vi "Vision_Left_R3.2.vi"() -> ()   [LabVIEW 2015]
uses:
  <vilib>/vision/Pattern Matching.llb/IMAQ Curve Parameters.ctl
  <vilib>/vision/Pattern Matching.llb/IMAQ Match Range Setting.ctl
  <vilib>/userdefined/High Color/IMAQdx.ctl
  <vilib>/vision/driver/NI_Vision_Acquisition_Software.lvlib
  <vilib>/vision/NI_Vision_Development_Module.lvlib
panel:
  in  "Range 0 Default\nSetting Values":T1={"Min Scale"=50.0, "Max Scale"=160.0, "Min Score"=850.0, "Lower Transition Scale"=55.0, "Upper Transition Scale"=200.0, "ROI Vertical"=4.5, "ROI Horizontal"=2.5, "Scale Cushion"=7.0, "Curve Parameters"={"Min Length"=20, "Row Search Step"=15, "Col Search Step"=15}, "Beacon Cushion (px)"=3.0, "Max Scale Diff\nfrom Main"=50.0}
  in  "Range 0 Templates":T2={"Sub - 2 File Path"=path "/home/lvuser/Beacon_Templates/Range_0/Range 0.png", "Sub Beacon Template File Path - ARRAY"=[path "/home/lvuser/Beacon_Templates/Range_1/Sub 0 - Range 1.png", path "/home/lvuser/Beacon_Templates/Range_1/Sub 1 - Range 1.png", path "/home/lvuser/Beacon_Templates/Range_1/Sub 2 - Range 1.png", path "/home/lvuser/Beacon_Templates/Range_1/Sub 3 - Range 1.png", path "/home/lvuser/Beacon_Templates/Range_1/Sub 4 - Range 1.png"]}
  in  "Correlation Score Threhsold (Range 0)":sgl=750.0
  in  "stop":bool
  in  "select (true= use advanced features\nfase= dont use)":bool
  in  "Range 3 Default\nSetting Values":T1={"Min Scale"=50.0, "Max Scale"=130.0, "Min Score"=800.0, "Lower Transition Scale"=1.0, "Upper Transition Scale"=120.0, "ROI Vertical"=3.5, "ROI Horizontal"=4.0, "Scale Cushion"=15.0, "Curve Parameters"={"Min Length"=2, "Row Search Step"=5, "Col Search Step"=5}, "Beacon Cushion (px)"=3.0, "Max Scale Diff\nfrom Main"=10.0}
  in  "Range 2 Default\nSetting Values":T1={"Min Scale"=75.0, "Max Scale"=130.0, "Min Score"=800.0, "Lower Transition Scale"=70.0, "Upper Transition Scale"=115.0, "ROI Vertical"=2.8, "ROI Horizontal"=4.0, "Scale Cushion"=17.0, "Curve Parameters"={"Min Length"=10, "Row Search Step"=10, "Col Search Step"=10}, "Beacon Cushion (px)"=7.0, "Max Scale Diff\nfrom Main"=20.0}
  in  "No Lock Default\nSetting Values":T3={"Min Scale"=25.0, "Max Scale"=125.0, "Min Score"=750.0, "Lower Transition Scale"=35.0, "Upper Transition Scale"=250.0, "ROI Vertical"=15.0, "ROI Horizontal"=15.0, "Scale Cushion"=15.0, "Curve Parameters"={"Min Length"=5, "Row Search Step"=10, "Col Search Step"=10}, "Scale Cushion 2"=15.0, "Max Scale Diff\nfrom Main"=15.0}
  in  "ROI Decay Factor (px)":dbl=50.0
  in  "ROBOT STATE\n(fwd, bwd, neither) 2":i32
  in  "Score Decay \nFactor 2":dbl=50.0
  in  "Range 1 Default\nSetting Values":T1={"Min Scale"=30.0, "Max Scale"=100.0, "Min Score"=800.0, "Lower Transition Scale"=35.0, "Upper Transition Scale"=67.0, "ROI Vertical"=0.75, "ROI Horizontal"=5.0, "Scale Cushion"=20.0, "Curve Parameters"={"Min Length"=15, "Row Search Step"=15, "Col Search Step"=15}, "Beacon Cushion (px)"=25.0, "Max Scale Diff\nfrom Main"=25.0}
  out "Next Template":T4(ring)=enum."Range 3"
  out "Current Template":T4(ring)=enum."Range 3"
  in  "Initial Template":T4(ring)
  in  "Range 3 Templates":T2={"Sub - 2 File Path"=path "/home/lvuser/Beacon_Templates/Range_3/5 Beacons - Range 3.png", "Sub Beacon Template File Path - ARRAY"=[path "/home/lvuser/Beacon_Templates/Range_3/Sub 0 - Range 3.png", path "/home/lvuser/Beacon_Templates/Range_3/Sub 1 - Range 3.png", path "/home/lvuser/Beacon_Templates/Range_3/Sub 2 - Range 3.png", path "/home/lvuser/Beacon_Templates/Range_3/Sub 3 - Range 3.png", path "/home/lvuser/Beacon_Templates/Range_3/Sub 4 - Range 3.png"]}
  in  "Range 2 Templates":T2={"Sub - 2 File Path"=path "/home/lvuser/Beacon_Templates/Range_2/5 Beacons - Range 2.png", "Sub Beacon Template File Path - ARRAY"=[path "/home/lvuser/Beacon_Templates/Range_2/Sub 0 - Range 2.png", path "/home/lvuser/Beacon_Templates/Range_2/Sub 1 - Range 2.png", path "/home/lvuser/Beacon_Templates/Range_2/Sub 2 - Range 2.png", path "/home/lvuser/Beacon_Templates/Range_2/Sub 3 - Range 2.png", path "/home/lvuser/Beacon_Templates/Range_2/Sub 4 - Range 2.png"]}
  in  "Range 1 Templates - LEFT":T2={"Sub - 2 File Path"=path "/home/lvuser/Beacon_Templates/Range_1/2_Beacons_Left - Range 1.png", "Sub Beacon Template File Path - ARRAY"=[path "/home/lvuser/Beacon_Templates/Range_1/Sub 0 - Range 1.png", path "/home/lvuser/Beacon_Templates/Range_1/Sub 1 - Range 1.png", path "/home/lvuser/Beacon_Templates/Range_1/Sub 2 - Range 1.png", path "/home/lvuser/Beacon_Templates/Range_1/Sub 3 - Range 1.png", path "/home/lvuser/Beacon_Templates/Range_1/Sub 4 - Range 1.png"]}
  out "Current Correlation Score":sgl=949.15265
  in  "Correlation Score Threhsold":sgl=300.0
  out "New Min Score":dbl=807.7509358723959
  out "New Low Scale":dbl=100.77034505208333
  out "New high Scale":dbl=130.77034505208331
  in  "Absolute\nMinimum Score":dbl=750.0
  in  "Absolute\nMaximum Scale":dbl=250.0
  in  "Absolute\nMinimum Scale":dbl=25.0
  in  "Score\nCushion":dbl=192.0
  in  "Avg Scale - Last":dbl=115.77034505208333
  in  "Avg Score - Last":dbl=999.7509358723959
  in  "Max Window\n for Avg":u8=3
  in  "Valid Treshold\nfor Lock":i16=3
  out "Current  Score":sgl=1000.0
  out "Current  Scale":sgl=115.65058
  out "Current Valid?":bool=TRUE
  out "Beacon - Scales":sgl[](array[numeric])=[104.281, 118.651344, 123.55058, 125.06095, 120.35953]
  out "beacon - Scores":sgl[](array[numeric])=[993.01056, 1000.0, 1000.0, 1000.0, 1000.0]
  out "Beacons Found":bool[](array[boolean])=[FALSE, TRUE, TRUE, TRUE, TRUE]
  out "Horiztonall Beacon \nCushion (pixels)":sgl=3.0
  out "Tracking Info":T5={"Lock"=TRUE, "Current Valid"=TRUE, "Current Template"=enum."Range 3", "Tracking Coordinates"={"X"=158.36672973632812, "Y"=119.79118347167969}, "Setting Values"={"Min Score"=807.7509358723959, "Min Scale"=100.77034505208333, "Max Scale"=130.77034505208331, "Curve Parameters"={"Min Length"=2, "Row Search Step"=5, "Col Search Step"=5}}}
  out "dT":u32=629
  out "Avg Scale":dbl=115.77034505208333
  out "Avg Score":dbl=999.7509358723959
  out "Current Search Settings":T8={"Curve Parameters"={"Extraction Mode"=1, "Edge Threshold"=200, "Edge Filter Size"=0, "Min Length"=2, "Row Search Step Size"=5, "Col Search Step Size"=5, "Max Endpoint Gap"=4, "Closed"=TRUE, "Subpixel"=TRUE}, "Match Mode"={"Rotation"=FALSE, "Scale"=TRUE, "Occlusion"=TRUE, "Reserved"=FALSE, "Reserved"=FALSE, "Reserved"=FALSE}, "Range Settings"=[{"Match Constraints"=0, "Min"=-2.0, "Max"=2.0}, {"Match Constraints"=1, "Min"=100.77034505208333, "Max"=130.77034505208331}, {"Match Constraints"=2, "Min"=0.0, "Max"=20.0}], "Number of Matches"=1, "Minimum Match Score"=807.7509, "SubPixel Accuracy"=TRUE, "Adv. Geometric Match Options 2"=[{"Setup Data Item"=20, "Item Value"=0.0}, {"Setup Data Item"=22, "Item Value"=1.0}]} {"Curve Parameters"."Extraction Mode" items=["Normal", "Uniform Regions"]; "Curve Parameters"."Edge Filter Size" items=["Fine", "Normal", "Contour Tracing"]; "Curve Parameters"."Max Endpoint Gap" min=0; "Curve Parameters"."Col Search Step Size" min=1 max=255 step=1; "Curve Parameters"."Row Search Step Size" min=1 max=255 step=1; "Curve Parameters"."Min Length" min=0; "Curve Parameters"."Edge Threshold" min=1 max=350 step=1; "Range Settings"."Max" format="%.2f"; "Range Settings"."Min" format="%.2f"; "Range Settings"."Match Constraints" items=["Rotation Angle (degrees)", "Scale Factor (%)", "Occlusion (%)"]}
  out "Valid Scale History":dbl[](array[numeric])=[115.65058135986328, 115.74882507324219, 111.08865356445312, 111.93978881835938, 115.91162872314453, 115.68242645263672, 115.45581817626953, 111.17475891113281, 111.21205139160156, 114.74717712402344, 114.64608001708984, 114.7938232421875, 116.48683166503906, 115.9120101928711, 114.3381576538086, 114.52978515625, 115.46134948730469, 116.78670501708984, 114.5467529296875] format="%#_13g"
  out "Valid Score History":dbl[](array[numeric])=[1000.0, 999.6264038085938, 991.4191284179688, 998.8792114257812, 999.6264038085938, 999.6264038085938, 1000.0, 991.4191284179688, 991.4191284179688, 1000.0, 1000.0, 1000.0, 1000.0, 996.72509765625, 1000.0, 1000.0, 1000.0, 1000.0, 1000.0] format="%#_13g"
  out "Valid Beacon History - in":bool[](array[boolean])=[TRUE, TRUE, FALSE, FALSE, TRUE, TRUE, TRUE, FALSE, FALSE, TRUE, FALSE, TRUE, TRUE, TRUE, TRUE, TRUE, TRUE, TRUE, TRUE]
  out "Startup Flag":bool
  out "Lock Status":bool=TRUE
  out "Y Coordinates":sgl[](array[numeric])=[118.2189, 119.13626, 119.99598, 121.06058, 122.42321]
  out "X Coordinates":sgl[](array[numeric])=[96.67693, 127.70059, 158.3874, 186.05737, 218.46037]
  out "Right Image out":T9(plugin-control)
  in  "History Size":i32=19
  in  "INITIAL Search Settings":T8={"Curve Parameters"={"Extraction Mode"=1, "Edge Threshold"=200, "Edge Filter Size"=0, "Min Length"=15, "Row Search Step Size"=10, "Col Search Step Size"=10, "Max Endpoint Gap"=4, "Closed"=TRUE, "Subpixel"=TRUE}, "Match Mode"={"Rotation"=FALSE, "Scale"=TRUE, "Occlusion"=TRUE, "Reserved"=FALSE, "Reserved"=FALSE, "Reserved"=FALSE}, "Range Settings"=[{"Match Constraints"=0, "Min"=-2.0, "Max"=2.0}, {"Match Constraints"=1, "Min"=25.0, "Max"=150.0}, {"Match Constraints"=2, "Min"=0.0, "Max"=20.0}], "Number of Matches"=1, "Minimum Match Score"=750.0, "SubPixel Accuracy"=TRUE, "Adv. Geometric Match Options 2"=[{"Setup Data Item"=20, "Item Value"=0.0}, {"Setup Data Item"=22, "Item Value"=1.0}]} {"Curve Parameters"."Extraction Mode" items=["Normal", "Uniform Regions"]; "Curve Parameters"."Edge Filter Size" items=["Fine", "Normal", "Contour Tracing"]; "Curve Parameters"."Max Endpoint Gap" min=0; "Curve Parameters"."Col Search Step Size" min=1 max=255 step=1; "Curve Parameters"."Row Search Step Size" min=1 max=255 step=1; "Curve Parameters"."Min Length" min=0; "Curve Parameters"."Edge Threshold" min=1 max=350 step=1; "Range Settings"."Max" format="%.2f"; "Range Settings"."Min" format="%.2f"; "Range Settings"."Match Constraints" items=["Rotation Angle (degrees)", "Scale Factor (%)", "Occlusion (%)"]; "Adv. Geometric Match Options 2"."Setup Data Item" items=["Curve Extraction Mode", "Curve Edge Threshold", "Curve Edge Filter Size", "Min Curve Length", "Curve Row Search Step Size", "Curve Col Search Step Size", "Curve Max Endpoint Gap", "Extract Closed Curves", "Enable Subpixel Curve Extraction", "Enable Correlation Score", "Enable Subpixel Accuracy", "Subpixel Iterations", "Subpixel Tolerance", "Initial Match List Length", "Enable Target Template Curve Score", "Min Match Separation Distance", "Min Match Separation Angle", "Min Match Separation Scale", "Max Match Overlap", "Enable Coarse Result", "Enable Calibration Support", "Enable Contrast Reversal", "Search Strategy", "Refinement Match Factor", "Subpixel Match Factor"]}
  # "ROI Factore (per Template)"
  # "Template Transition Scales"
  # "Search Parameter Limits"
  # "TEMPLATE FILE PATHS"
  # "Config"
  # "Initial Settings"
  # "Range"
  # "Range"
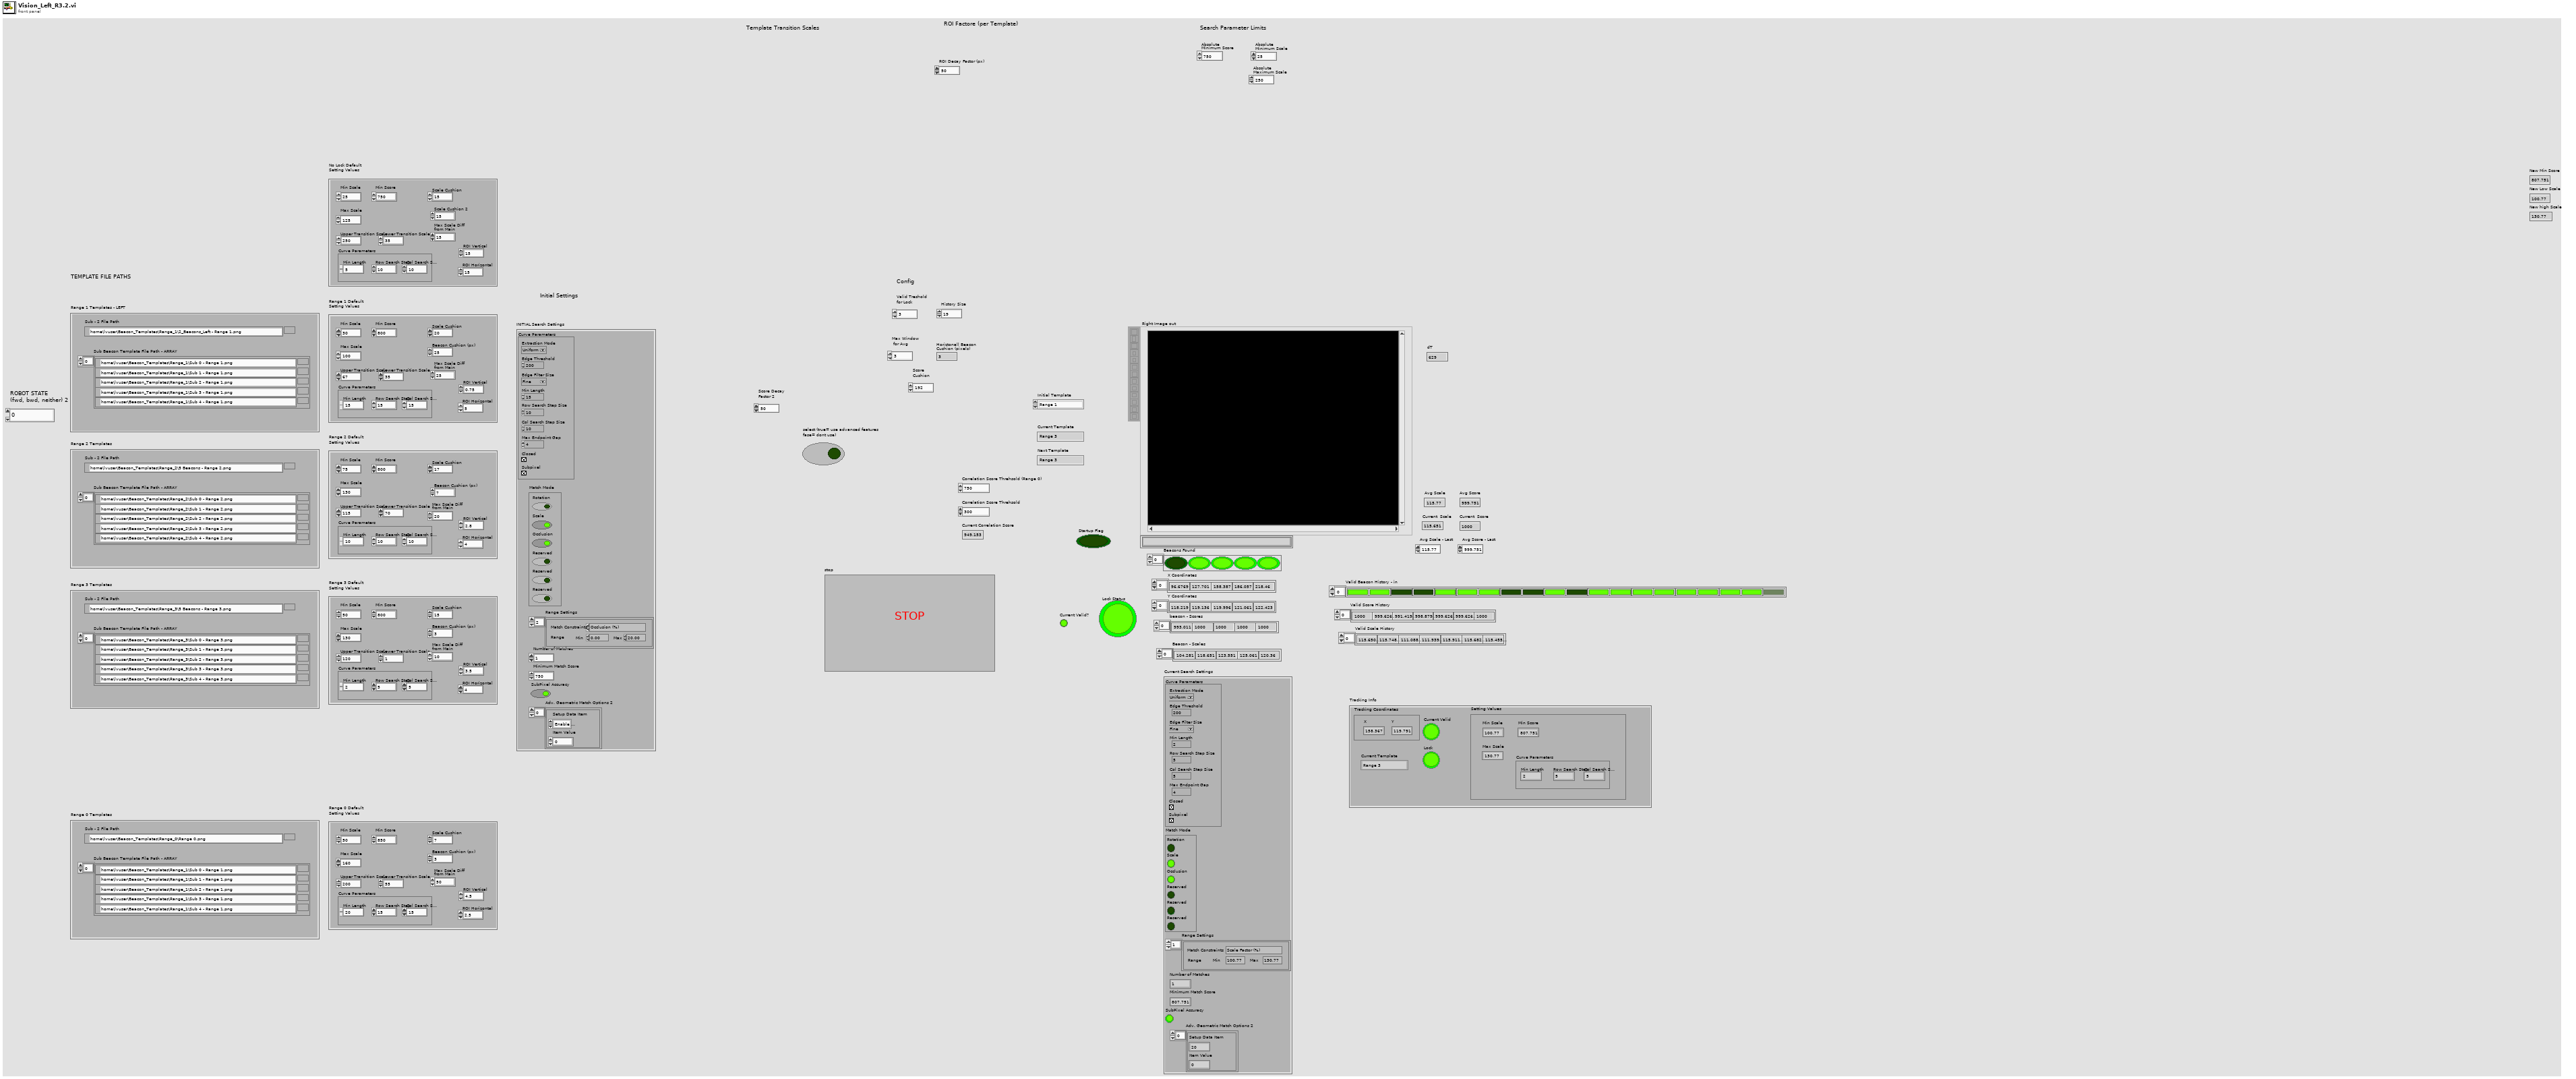
[diagram p1: front panel]
types:
  T1 = cluster{"Min Scale":dbl, "Max Scale":dbl, "Min Score":dbl, "Lower Transition Scale":sgl, "Upper Transition Scale":sgl, "ROI Vertical":dbl, "ROI Horizontal":dbl, "Scale Cushion":dbl, "Curve Parameters":cluster{"Min Length":i32, "Row Search Step":i32, "Col Search Step":i32}, "Beacon Cushion (px)":dbl, "Max Scale Diff\nfrom Main":dbl}
  T2 = cluster{"Sub - 2 File Path":path, "Sub Beacon Template File Path - ARRAY":path[]}
  T3 = cluster{"Min Scale":dbl, "Max Scale":dbl, "Min Score":dbl, "Lower Transition Scale":sgl, "Upper Transition Scale":sgl, "ROI Vertical":dbl, "ROI Horizontal":dbl, "Scale Cushion":dbl, "Curve Parameters":cluster{"Min Length":i32, "Row Search Step":i32, "Col Search Step":i32}, "Scale Cushion 2":dbl, "Max Scale Diff\nfrom Main":dbl}
  T4 = enum16{"Range 1", "Range 2", "Range 3", "Range 0"}
  T5 = cluster{"Lock":bool, "Current Valid":bool, "Current Template":enum16{"Range 1", "Range 2", "Range 3", "Range 0"}, "Tracking Coordinates":cluster{"X":dbl, "Y":dbl}, "Setting Values":cluster{"Min Score":dbl, "Min Scale":dbl, "Max Scale":dbl, "Curve Parameters":cluster{"Min Length":i32, "Row Search Step":i32, "Col Search Step":i32}}}
  T6 = typedef "IMAQ Curve Parameters.ctl" = cluster{"Extraction Mode":u32, "Edge Threshold":i32, "Edge Filter Size":u32, "Min Length":i32, "Row Search Step Size":i32, "Col Search Step Size":i32, "Max Endpoint Gap":i32, "Closed":bool, "Subpixel":bool}
  T7 = typedef "IMAQ Match Range Setting.ctl" = cluster{"Match Constraints":u32, "Min":dbl, "Max":dbl}
  T8 = cluster{"Curve Parameters":T6, "Match Mode":cluster{"Rotation":bool, "Scale":bool, "Occlusion":bool, "Reserved":bool, "Reserved":bool, "Reserved":bool}, "Range Settings":T7[], "Number of Matches":i32, "Minimum Match Score":sgl, "SubPixel Accuracy":bool, "Adv. Geometric Match Options 2":cluster{"Setup Data Item":u16, "Item Value":dbl}[]}
  T9 = typedef "IMAQ Image.ctl" = refnum<image>
  T10 = typedef "IMAQdx.ctl" = refnum<k21>
  T11 = typedef "Image Type" = u32
  T12 = typedef "ROI Descriptor" = cluster{"Global Rectangle":i32[], "Contours":cluster{"ID":enum32{"External", "Internal"}, "Type":u32, "Coordinates":i32[]}[]}
  T13 = typedef "IMAQ GM Match Report.ctl" = cluster{"Position":cluster{"x":sgl, "y":sgl}, "Angle":sgl, "Scale":sgl, "Score":sgl, "Bounding Box":cluster{"x":sgl, "y":sgl}[], "Contrast Reversed":bool, "Occlusion %":sgl, "Template Target Curve Score":sgl, "Target Template Curve Score":sgl, "Correlation Score":sgl}
  T14 = cluster{"Matches[0]":T13, "Matches[1]":T13, "Matches[2]":T13, "Matches[3]":T13, "Matches[4]":T13, "Matches[5]":T13, "Matches[6]":T13, "Matches[7]":T13, "Matches[8]":T13}
  T15 = cluster{"Bounding Box[0]":cluster{"x":sgl, "y":sgl}, "Bounding Box[1]":cluster{"x":sgl, "y":sgl}, "Bounding Box[2]":cluster{"x":sgl, "y":sgl}, "Bounding Box[3]":cluster{"x":sgl, "y":sgl}, "Bounding Box[4]":cluster{"x":sgl, "y":sgl}, "Bounding Box[5]":cluster{"x":sgl, "y":sgl}, "Bounding Box[6]":cluster{"x":sgl, "y":sgl}, "Bounding Box[7]":cluster{"x":sgl, "y":sgl}, "Bounding Box[8]":cluster{"x":sgl, "y":sgl}}
  T16 = cluster{"Matches (Geometric Matching 1)[0]":T13, "Matches (Geometric Matching 1)[1]":T13, "Matches (Geometric Matching 1)[2]":T13, "Matches (Geometric Matching 1)[3]":T13, "Matches (Geometric Matching 1)[4]":T13, "Matches (Geometric Matching 1)[5]":T13, "Matches (Geometric Matching 1)[6]":T13, "Matches (Geometric Matching 1)[7]":T13, "Matches (Geometric Matching 1)[8]":T13}
  T17 = cluster{"Min Length":i32, "Row Search Step":i32, "Col Search Step":i32}
  T18 = cluster{"Extraction Mode":u32, "Edge Threshold":i32, "Edge Filter Size":u32, "Min Length":i32, "Row Search Step":i32, "Col Search Step":i32, "Max Endpoint Gap":i32, "Closed":bool, "Subpixel":bool}
  T19 = typedef "IMAQ Rectangle" = cluster{"Left":i32, "Top":i32, "Right":i32, "Bottom":i32, "Rotation":dbl}
  T20 = cluster{"Min Length":i32, "Row Search Step Size":i32, "Col Search Step Size":i32}
  T21 = cluster{"Min Score":dbl, "Min":dbl, "Max":dbl, cluster{"Min Length":i32, "Row Search Step Size":i32, "Col Search Step Size":i32}}
  T22 = cluster{bool, bool, "Initial Template":enum16{"Range 1", "Range 2", "Range 3", "Range 0"}, "Position":cluster{"x":dbl, "y":dbl}, cluster{"Min Score":dbl, "Min":dbl, "Max":dbl, cluster{"Min Length":i32, "Row Search Step Size":i32, "Col Search Step Size":i32}}}
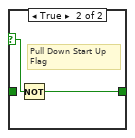
[diagram p2: hidden frame]
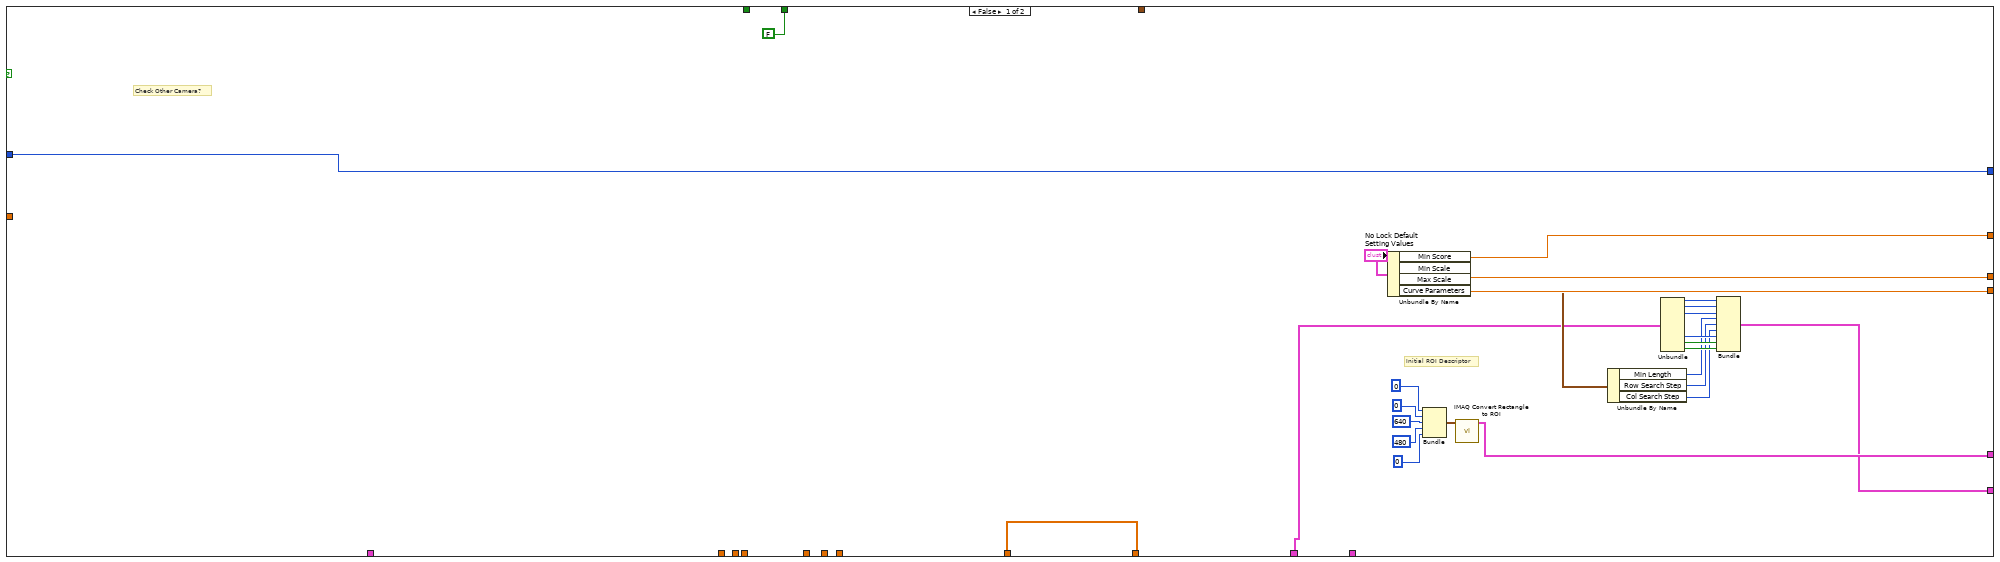
[diagram p3: hidden frame]
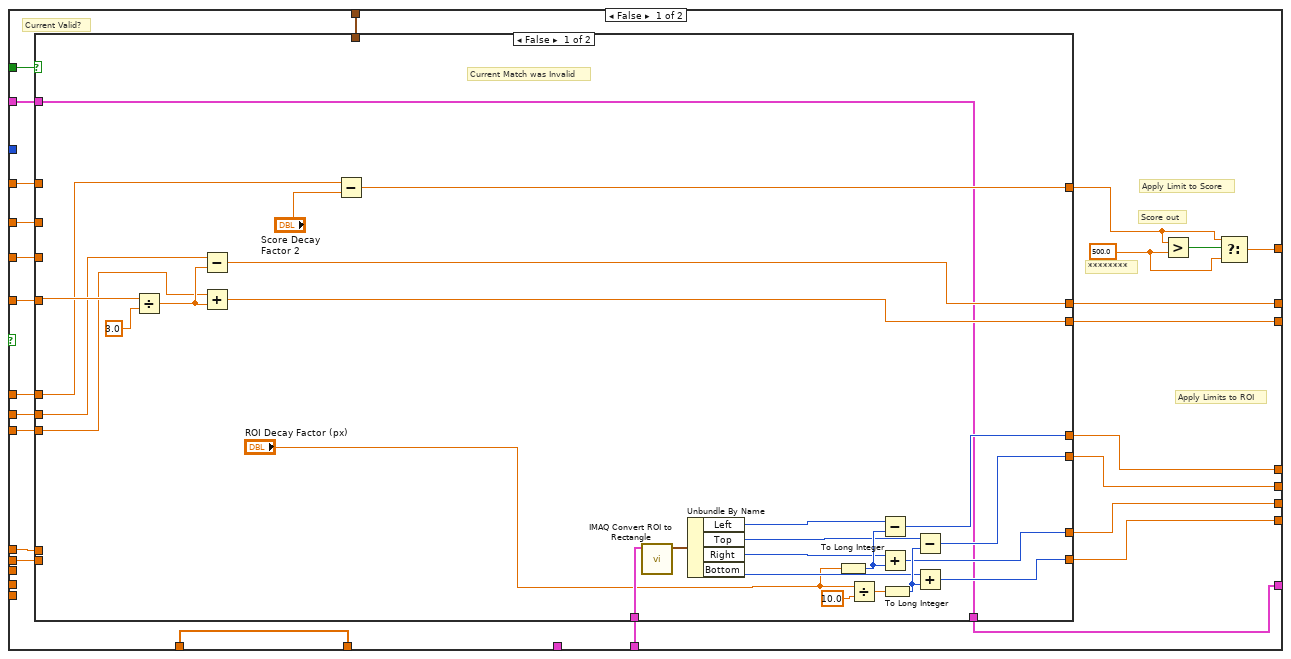
[diagram p4: hidden frame]
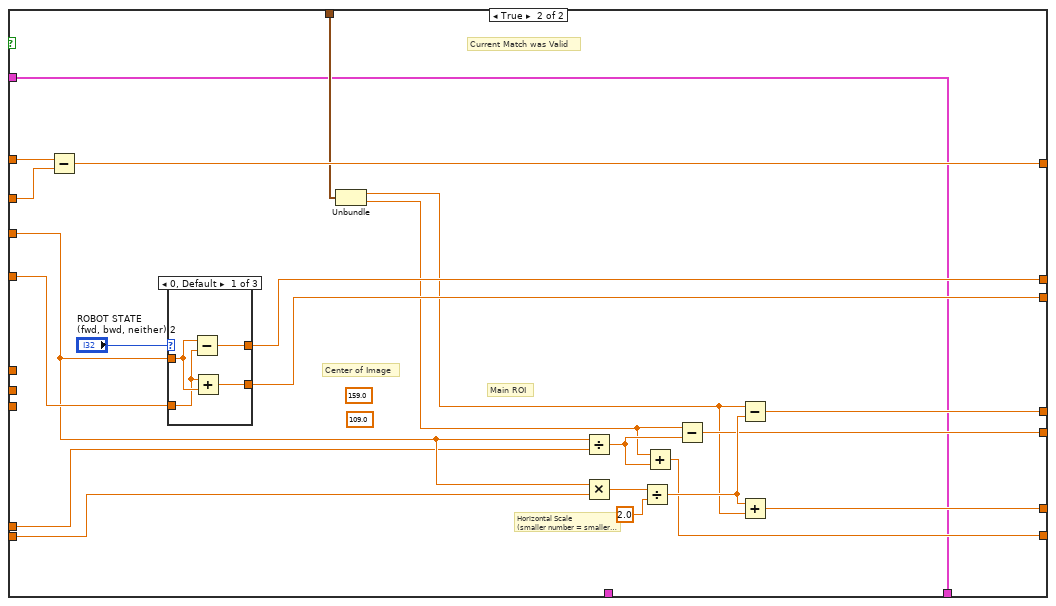
[diagram p5: hidden frame]
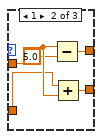
[diagram p6: hidden frame]
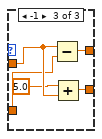
[diagram p7: hidden frame]
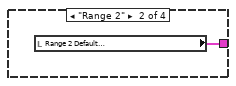
[diagram p8: hidden frame]
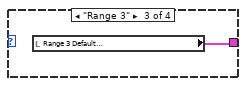
[diagram p9: hidden frame]
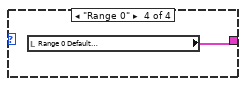
[diagram p10: hidden frame]
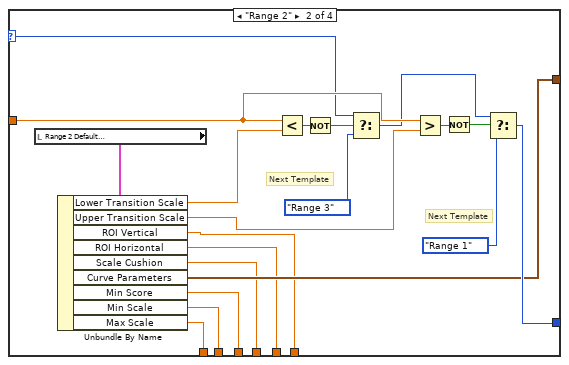
[diagram p11: hidden frame]
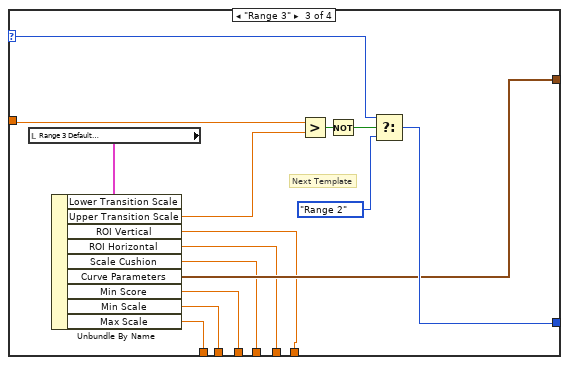
[diagram p12: hidden frame]
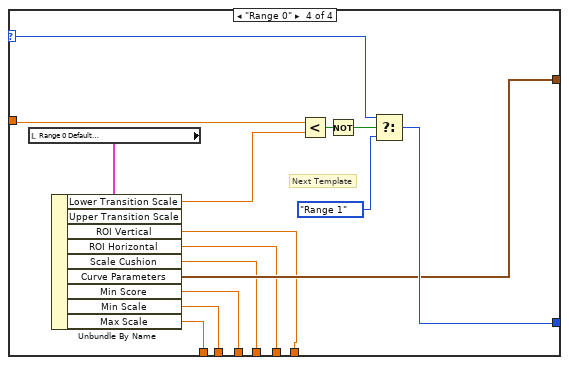
[diagram p13: hidden frame]
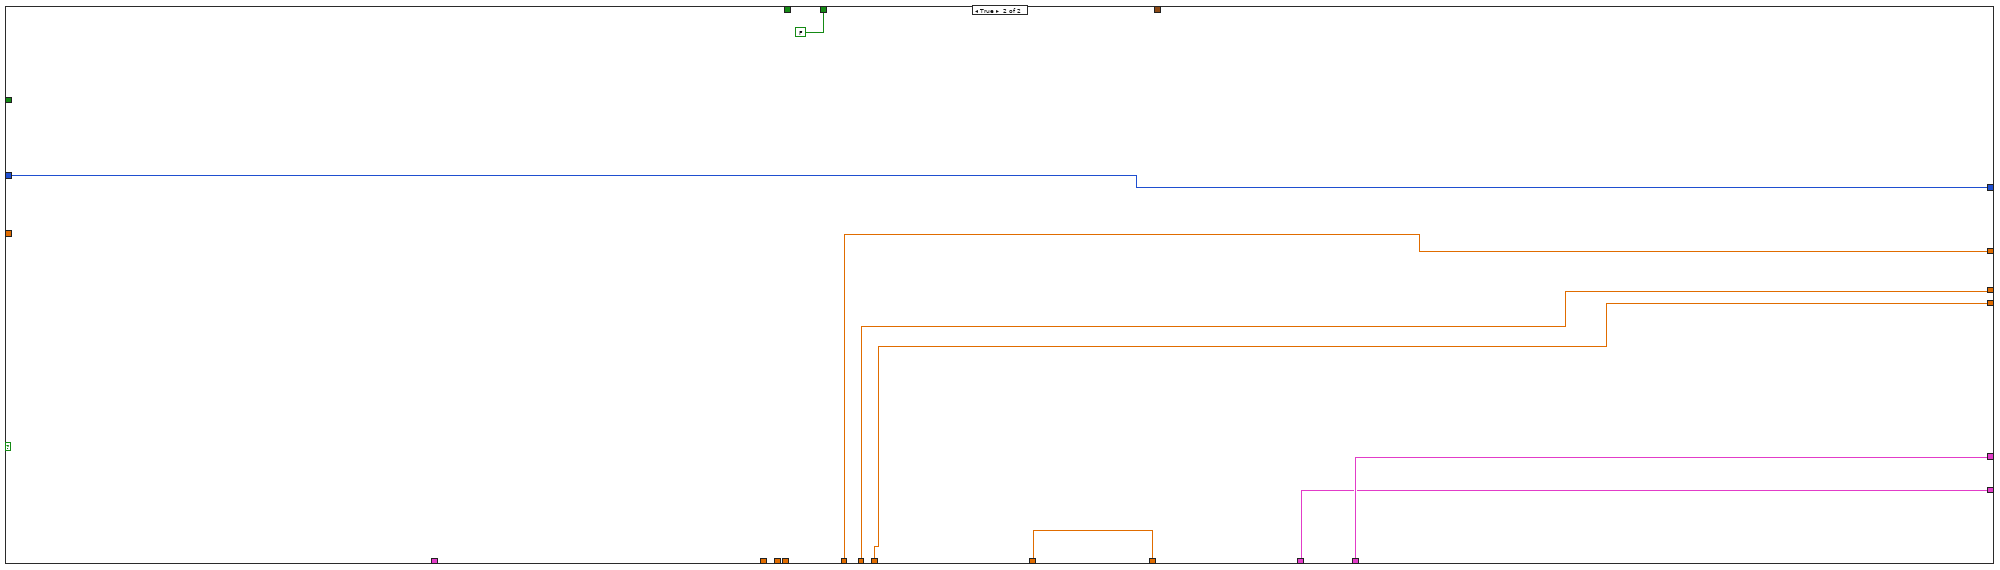
[diagram p14: hidden frame]
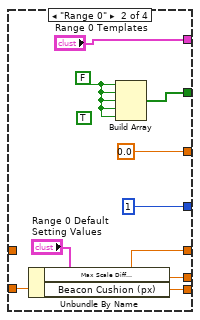
[diagram p15: hidden frame]
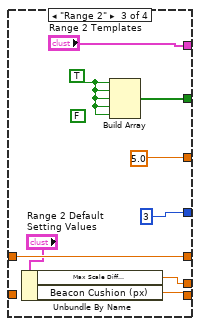
[diagram p16: hidden frame]
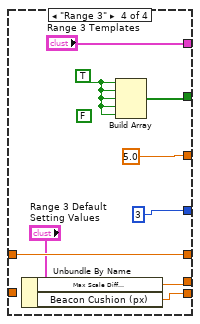
[diagram p17: hidden frame]
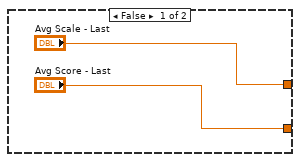
[diagram p18: hidden frame]
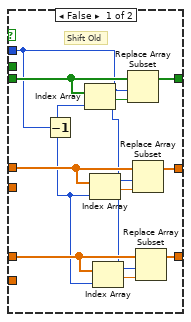
[diagram p20: hidden frame]
diagram:
  n1 = flat-sequence {
    tunnel: [w38] -> w16
    tunnel: ["INITIAL Search Settings"] -> w15
    tunnel: ["Initial Template"] -> w14
    tunnel: [TRUE] -> w13
    tunnel: [w35] -> w12
    tunnel: [w34] -> w11
    tunnel: [w33] -> w10
    tunnel: [w32] -> w9
    tunnel: [w31] -> w8
    tunnel: ["History Size"] -> w7
    tunnel: [750.0] -> w6
    tunnel: [100.0] -> w5
    tunnel: [w19] -> w4
    tunnel: [w18] -> w3
    tunnel: [w17] -> w2
    tunnel: w16 -> [w64]
    tunnel: w15 -> [w63]
    tunnel: w14 -> [w62]
    tunnel: w13 -> [w61]
    tunnel: w12 -> [w57]
    tunnel: w11 -> [w54]
    tunnel: w10 -> [w60]
    tunnel: w9 -> [w59]
    tunnel: w8 -> [w58]
    tunnel: w7 -> [w56]
    tunnel: w6 -> [_]
    tunnel: w5 -> [_]
    tunnel: w4 -> [w53]
    tunnel: w3 -> [w52]
    tunnel: w2 -> [w51]
    tunnel: [w50] -> w1
    tunnel: w1 -> [w830]
    frame #0 {
      w24 = "[NIIMAQ_HEADER]\nType = 2\nVersion = 8\n\n[CAMERA_DATA]\nAcquisitionAttributes::Bayer::Algorithm = \"Bilinear\"\nAcquisitionAttributes::Bayer::GainB = \"1\"\nAcquisitionAttributes::Bayer::GainG = \"1\"\nAcquisitionAttributes::Bayer::GainR = \"1\"\nAcquisitionAttributes::Bayer::Pattern = \"Use hardware value\"\nAcquisitionAttributes::BitsPerPixel = \"Use hardware value\"\nAcquisitionAttributes::IgnoreFirstFrame = \"false\"\nAcquisitionAttributes::ImageDecoderCopyMode = \"Auto\"\nAcquisitionAttributes::OutputImageType = \"Auto\"\nAcquisitionAttributes::OverwriteMode = \"Get Newest\"\nAcquisitionAttributes::PixelSignedness = \"Use hardware value\"\nAcquisitionAttributes::ReceiveTimestampMode = \"None\"\nAcquisitionAttributes::ShiftPixelBits = \"false\"\nAcquisitionAttributes::SwapPixelBytes = \"false\"\nAcquisitionAttributes::Timeout = \"5000\"\nAcquisitionAttributes::VerticalMirror = \"false\"\nAcquisitionAttributes::VideoMode = \"320x240 YUY2 30.00fps\"\nCameraAttributes::BacklightCompensation::Mode = \"Manual\"\nCameraAttributes::BacklightCompensation::Value = \"false\"\nCameraAttributes::Brightness::Mode = \"UnknownEnumValue\"\nCameraAttributes::Brightness::Value = \"133\"\nCameraAttributes::Contrast::Mode = \"Manual\"\nCameraAttributes::Contrast::Value = \"0\"\nCameraAttributes::Exposure::Mode = \"Auto\"\nCameraAttributes::Focus::Mode = \"Auto\"\nCameraAttributes::Pan::Mode = \"Manual\"\nCameraAttributes::Pan::Value = \"0\"\nCameraAttributes::Saturation::Mode = \"Manual\"\nCameraAttributes::Saturation::Value = \"103\"\nCameraAttributes::Sharpness::Mode = \"Manual\"\nCameraAttributes::Sharpness::Value = \"25\"\nCameraAttributes::Tilt::Mode = \"Manual\"\nCameraAttributes::Tilt::Value = \"0\"\nCameraAttributes::WhiteBalance::Mode = \"Auto\"\nCameraAttributes::Zoom::Mode = \"Manual\"\nCameraAttributes::Zoom::Value = \"0\"\n"  # Attributes
      w45 = T11 0 items=["Grayscale (U8)", "Grayscale (I16)", "Grayscale (SGL)", "Complex (CSG)", "RGB (U32)", "HSL (U32)", "RGB (U64)", "Grayscale (U16)"] ("Image Type")
      # "avg start scale"
      # "Score History"
      # "Scale History"
      # "Valid Match History\n(main beacon)"
      # "Template State"
      # "Search Parameters"
      # "StartUp = True"
      # "Initial ROI Descriptor"
      # "INITIALIZE"
      n2 = call <vilib>:"IMAQdx Open Camera.vi"("Session In"=T10 "cam0") -> ("error out"=w22:errorcluster, "Session Out"=w23:T10)  [unwired: 2 in, 7 out]
      n3 = call <vilib>:"IMAQdx Read Attributes From String.vi"("error in"=w22, "Attributes String In"=w24, "Session In"=w23) -> ("error out"=w21:errorcluster, "Session Out"=w20:T10)  [unwired: 7 out]
      n4 = Bundle(0, 0, 640, 480, 0) -> (w44:cluster{i32, i32, i32, i32, i32})  [unwired: 1 in]
      n5 = call "IMAQ Convert Rectangle to ROI"("Rectangle"=w44) -> ("ROI Descriptor"=w38:T12)  [unwired: 8 in, 1 out]
      n6 = call "IMAQ Create"("Image Name"="Left_Image", "Image Type"=w45) -> ("New Image"=w35:T9, "error out"=w34:errorcluster)  [unwired: 3 in]
      n7 = Initialize Array(FALSE, "History Size") -> (w33:bool[])
      n8 = Initialize Array(0.0, "History Size") -> (w31:dbl[])
      n9 = Initialize Array(0.0, "History Size") -> (w32:dbl[])
      n10 = call <vilib>:"IMAQdx Configure Grab.vi"("error in"=w21, "Session In"=w20) -> ("error out"=w17:errorcluster, "Session Out"=w19:T10)  [unwired: 8 in]
      n11 = call "IMAQ Create"("Image Name"="Original") -> ("New Image"=w18:T9)  [unwired: 4 in, 1 out]
    }
    frame #1 {
      # "Avg Scale"
      # "Avg Score"
      # "Score History"
      # "Scale History"
      # "Valid Match History\n(main beacon)"
      # "Sub Beacon Search Array"
      # "StartUp = True"
      # "Template State"
      # "Search Parameters"
      # "ROI"
      n12 = call "Tick Count"() -> ("Tick Count(mSec)"=w55:u32)
      n13 = while {
        shift-right: [w77] -> _
        shift-left: w64 -> [w91]
        shift-right: [w87] -> _
        shift-left: w63 -> [w92]
        shift-right: [w76] -> _
        shift-left: w62 -> [w79]
        shift-right: [w74] -> _
        shift-left: w61 -> [w75]
        shift-right: [w83] -> _
        shift-left: w60 -> [w84]
        shift-right: [w73] -> _
        shift-left: w59 -> [w82]
        shift-right: [w80] -> _
        shift-left: w58 -> [w81]
        shift-right: [w86] -> _
        shift-left: w57 -> [w93]
        tunnel: w56 -> [w98]
        shift-right: [w96] -> _
        shift-left: w55 -> [w97]
        tunnel: w54 -> [w85]
        tunnel: w53 -> [w72]
        tunnel: w52 -> [w71]
        tunnel: w51 -> [w70]
        tunnel: [w67] -> w50
        stop <- "stop" stop-if-true
        n14 = call "Tick Count2"() -> ("Tick Count(mSec)"=w96:u32)
        n15 = Subtract(x=w96, y=w97) -> (x-y=→"dT":u32)
        n16 = flat-sequence {
          tunnel: [w106] -> w89
          tunnel: [w105] -> w94
          tunnel: w93 -> [w105]
          tunnel: [w105] -> w86
          tunnel: w85 -> [_]
          tunnel: w72 -> [w104]
          tunnel: w71 -> [w103]
          tunnel: w70 -> [w102]
          tunnel: [w101] -> w69
          tunnel: [w100] -> w68
          tunnel: [w99] -> w66
          tunnel: w79 -> [w111]
          tunnel: w84 -> [w224]
          tunnel: w82 -> [w223]
          tunnel: w81 -> [w222]
          tunnel: w98 -> [_]
          tunnel: w94 -> [w122]
          tunnel: w92 -> [w123]
          tunnel: w91 -> [w125]
          tunnel: [w191] -> w90
          tunnel: w89 -> [w180]
          tunnel: [w180] -> w88
          tunnel: [w179] -> w83
          tunnel: [w147] -> _
          tunnel: [w178] -> w80
          tunnel: w75 -> [w144]
          tunnel: [w149] -> w78
          tunnel: [w150] -> w77
          tunnel: [w149] -> w76
          tunnel: [w143] -> w74
          tunnel: [w148] -> w73
          tunnel: w69 -> [w117]
          tunnel: w68 -> [w116]
          tunnel: [w115] -> w67
          tunnel: w66 -> [w115]
          tunnel: w90 -> [w827]
          tunnel: w88 -> [w828]
          tunnel: [w827] -> w87
          tunnel: [w826] -> _
          tunnel: w78 -> [w826]
          frame #0 {
            # "Aquire Image"
            n17 = shared-variable "RT myRIO Target - Overlord\\Localization_Variables_r0.lvlib\\Left Servo Angle_Current"() -> (w106:dbl)  [unwired: 1 in, 1 out]
            n18 = call <vilib>:"IMAQdx Grab2.vi"("error in"=w102, "Image In"=w103, "Session In"=w104) -> ("error out"=w100:errorcluster, "Image Out"=w101:T9, "Session Out"=w99:T10)  [unwired: 5 in, 1 out]
          }
          frame #1 {
            (unwired) T4."Range 1" ("Initial Template 2")
            w135 = 6 items=["Red", "Green", "Blue", "Hue", "Saturation", "Luminance", "Value", "Intensity"] ("Color Plane")
            w194 = u32 1 ("index")
            # "Tracking Position"
            # "ROI center"
            # "Add mode when CLose to look for all individual beacons with full ROI"
            # "Service Start Up Flag"
            # "Change States?"
            # "Next Template"
            # "Max Scale"
            # "Min Scale"
            # "Min Score"
            # "Curve p"
            # "ROI"
            # "Current Scale Range"
            # "Current Min Score"
            # "Avg Score"
            # "Avg Scale"
            # "Startup?"
            # "********** Look into False case **********"
            # "SUm # of Sub-Beacons Found, Check if Enoough\nto be considered Valid"
            # "Update Tracking Coordinates"
            # "Next Settings"
            # "Current Settings"
            # "Current Min\n& Max Scale"
            # "Scale"
            # "Min Score"
            # "Lower Scale"
            # "Upper Scale"
            # "Min Score out"
            # "Score History"
            # "Min Required to use avarage"
            # "Scale History"
            # "History Size"
            # "Calculate Average Score/Scale"
            # "****# of previous in history that must be true\nin order for position to be considered \"locked\""
            # "Scale History"
            # "Score History"
            # "Valid History"
            # "Update History Data"
            # "1 Match FOund?"
            # "# of Sub Beacons"
            # "Sub Beacons to Search For"
            # "# Sub Beacons to Find in\norder to be valid"
            # "Template Filepath & Sub Beacon Array"
            # "Select Current Template Config"
            # "Pattern Match to Current Template"
            # "Apply FIltering"
            n19 = call "IMAQ ImageBorderSize"("Get/Set Status? (Set)"=TRUE, "Image"=w117, "Image border size in"=13 ("Border Size"), "error in (no error)"=w116) -> ("Image Out"=w134:T9, "error out"=w138:errorcluster)  [unwired: 1 out]
            n20 = call "IMAQ ExtractSingleColorPlane"("Color Plane"=w135, "error in (no error)"=w138, "Image Src"=w134) -> ("error out"=w133:errorcluster, "Image Dst Out"=w131:T9)  [unwired: 1 in, 6 out]
            n21 = call "IMAQ Convolute"("Kernel"=sgl[][] [[1.0, 2.0, 1.0], [2.0, 4.0, 2.0], [1.0, 2.0, 1.0]], "Divider (kernel sum)"=sgl 9.0 ("Divider"), "error in (no error)"=w133, "Image Src"=w131) -> ("error out"=w130:errorcluster, "Image Dst Out"=w127:T9)  [unwired: 3 in, 3 out]
            n22 = call "IMAQ Convolute"("Kernel"=sgl[][] [[-1.0, -1.0, -1.0, -1.0, -1.0, -1.0, -1.0, -1.0, -1.0, -1.0, -1.0, -1.0, -1.0, -1.0, -1.0, -1.0, -1.0, -1.0, -1.0, -1.0, -1.0, -1.0, -1.0, -1.0, -1.0, -1.0, -1.0], [-1.0, -1.0, -1.0, -1.0, -1.0, -1.0, -1.0, -1.0, -1.0, -1.0, -1.0, -1.0, -1.0, -1.0, -1.0, -1.0, -1.0, -1.0, -1.0, -1.0, -1.0, -1.0, -1.0, -1.0, -1.0, -1.0, -1.0], [-1.0, -1.0, -1.0, -1.0, -1.0, -1.0, -1.0, -1.0, -1.0, -1.0, -1.0, -1.0, -1.0, -1.0, -1.0, -1.0, -1.0, -1.0, -1.0, -1.0, -1.0, -1.0, -1.0, -1.0, -1.0, -1.0, -1.0], [-1.0, -1.0, -1.0, -1.0, -1.0, -1.0, -1.0, -1.0, -1.0, -1.0, -1.0, -1.0, -1.0, -1.0, -1.0, -1.0, -1.0, -1.0, -1.0, -1.0, -1.0, -1.0, -1.0, -1.0, -1.0, -1.0, -1.0], [-1.0, -1.0, -1.0, -1.0, -1.0, -1.0, -1.0, -1.0, -1.0, -1.0, -1.0, -1.0, -1.0, -1.0, -1.0, -1.0, -1.0, -1.0, -1.0, -1.0, -1.0, -1.0, -1.0, -1.0, -1.0, -1.0, -1.0], [-1.0, -1.0, -1.0, -1.0, -1.0, -1.0, -1.0, -1.0, -1.0, -1.0, -1.0, -1.0, -1.0, -1.0, -1.0, -1.0, -1.0, -1.0, -1.0, -1.0, -1.0, -1.0, -1.0, -1.0, -1.0, -1.0, -1.0], [-1.0, -1.0, -1.0, -1.0, -1.0, -1.0, -1.0, -1.0, -1.0, -1.0, -1.0, -1.0, -1.0, -1.0, -1.0, -1.0, -1.0, -1.0, -1.0, -1.0, -1.0, -1.0, -1.0, -1.0, -1.0, -1.0, -1.0], [-1.0, -1.0, -1.0, -1.0, -1.0, -1.0, -1.0, -1.0, -1.0, -1.0, -1.0, -1.0, -1.0, -1.0, -1.0, -1.0, -1.0, -1.0, -1.0, -1.0, -1.0, -1.0, -1.0, -1.0, -1.0, -1.0, -1.0], [-1.0, -1.0, -1.0, -1.0, -1.0, -1.0, -1.0, -1.0, -1.0, -1.0, -1.0, -1.0, -1.0, -1.0, -1.0, -1.0, -1.0, -1.0, -1.0, -1.0, -1.0, -1.0, -1.0, -1.0, -1.0, -1.0, -1.0], [-1.0, -1.0, -1.0, -1.0, -1.0, -1.0, -1.0, -1.0, -1.0, -1.0, -1.0, -1.0, -1.0, -1.0, -1.0, -1.0, -1.0, -1.0, -1.0, -1.0, -1.0, -1.0, -1.0, -1.0, -1.0, -1.0, -1.0], [-1.0, -1.0, -1.0, -1.0, -1.0, -1.0, -1.0, -1.0, -1.0, -1.0, -1.0, -1.0, -1.0, -1.0, -1.0, -1.0, -1.0, -1.0, -1.0, -1.0, -1.0, -1.0, -1.0, -1.0, -1.0, -1.0, -1.0], [-1.0, -1.0, -1.0, -1.0, -1.0, -1.0, -1.0, -1.0, -1.0, -1.0, -1.0, -1.0, -1.0, -1.0, -1.0, -1.0, -1.0, -1.0, -1.0, -1.0, -1.0, -1.0, -1.0, -1.0, -1.0, -1.0, -1.0], [-1.0, -1.0, -1.0, -1.0, -1.0, -1.0, -1.0, -1.0, -1.0, -1.0, -1.0, -1.0, -1.0, -1.0, -1.0, -1.0, -1.0, -1.0, -1.0, -1.0, -1.0, -1.0, -1.0, -1.0, -1.0, -1.0, -1.0], [-1.0, -1.0, -1.0, -1.0, -1.0, -1.0, -1.0, -1.0, -1.0, -1.0, -1.0, -1.0, -1.0, 728.0, -1.0, -1.0, -1.0, -1.0, -1.0, -1.0, -1.0, -1.0, -1.0, -1.0, -1.0, -1.0, -1.0], [-1.0, -1.0, -1.0, -1.0, -1.0, -1.0, -1.0, -1.0, -1.0, -1.0, -1.0, -1.0, -1.0, -1.0, -1.0, -1.0, -1.0, -1.0, -1.0, -1.0, -1.0, -1.0, -1.0, -1.0, -1.0, -1.0, -1.0], [-1.0, -1.0, -1.0, -1.0, -1.0, -1.0, -1.0, -1.0, -1.0, -1.0, -1.0, -1.0, -1.0, -1.0, -1.0, -1.0, -1.0, -1.0, -1.0, -1.0, -1.0, -1.0, -1.0, -1.0, -1.0, -1.0, -1.0], [-1.0, -1.0, -1.0, -1.0, -1.0, -1.0, -1.0, -1.0, -1.0, -1.0, -1.0, -1.0, -1.0, -1.0, -1.0, -1.0, -1.0, -1.0, -1.0, -1.0, -1.0, -1.0, -1.0, -1.0, -1.0, -1.0, -1.0], [-1.0, -1.0, -1.0, -1.0, -1.0, -1.0, -1.0, -1.0, -1.0, -1.0, -1.0, -1.0, -1.0, -1.0, -1.0, -1.0, -1.0, -1.0, -1.0, -1.0, -1.0, -1.0, -1.0, -1.0, -1.0, -1.0, -1.0], [-1.0, -1.0, -1.0, -1.0, -1.0, -1.0, -1.0, -1.0, -1.0, -1.0, -1.0, -1.0, -1.0, -1.0, -1.0, -1.0, -1.0, -1.0, -1.0, -1.0, -1.0, -1.0, -1.0, -1.0, -1.0, -1.0, -1.0], [-1.0, -1.0, -1.0, -1.0, -1.0, -1.0, -1.0, -1.0, -1.0, -1.0, -1.0, -1.0, -1.0, -1.0, -1.0, -1.0, -1.0, -1.0, -1.0, -1.0, -1.0, -1.0, -1.0, -1.0, -1.0, -1.0, -1.0], [-1.0, -1.0, -1.0, -1.0, -1.0, -1.0, -1.0, -1.0, -1.0, -1.0, -1.0, -1.0, -1.0, -1.0, -1.0, -1.0, -1.0, -1.0, -1.0, -1.0, -1.0, -1.0, -1.0, -1.0, -1.0, -1.0, -1.0], [-1.0, -1.0, -1.0, -1.0, -1.0, -1.0, -1.0, -1.0, -1.0, -1.0, -1.0, -1.0, -1.0, -1.0, -1.0, -1.0, -1.0, -1.0, -1.0, -1.0, -1.0, -1.0, -1.0, -1.0, -1.0, -1.0, -1.0], [-1.0, -1.0, -1.0, -1.0, -1.0, -1.0, -1.0, -1.0, -1.0, -1.0, -1.0, -1.0, -1.0, -1.0, -1.0, -1.0, -1.0, -1.0, -1.0, -1.0, -1.0, -1.0, -1.0, -1.0, -1.0, -1.0, -1.0], [-1.0, -1.0, -1.0, -1.0, -1.0, -1.0, -1.0, -1.0, -1.0, -1.0, -1.0, -1.0, -1.0, -1.0, -1.0, -1.0, -1.0, -1.0, -1.0, -1.0, -1.0, -1.0, -1.0, -1.0, -1.0, -1.0, -1.0], [-1.0, -1.0, -1.0, -1.0, -1.0, -1.0, -1.0, -1.0, -1.0, -1.0, -1.0, -1.0, -1.0, -1.0, -1.0, -1.0, -1.0, -1.0, -1.0, -1.0, -1.0, -1.0, -1.0, -1.0, -1.0, -1.0, -1.0], [-1.0, -1.0, -1.0, -1.0, -1.0, -1.0, -1.0, -1.0, -1.0, -1.0, -1.0, -1.0, -1.0, -1.0, -1.0, -1.0, -1.0, -1.0, -1.0, -1.0, -1.0, -1.0, -1.0, -1.0, -1.0, -1.0, -1.0], [-1.0, -1.0, -1.0, -1.0, -1.0, -1.0, -1.0, -1.0, -1.0, -1.0, -1.0, -1.0, -1.0, -1.0, -1.0, -1.0, -1.0, -1.0, -1.0, -1.0, -1.0, -1.0, -1.0, -1.0, -1.0, -1.0, -1.0]], "Divider (kernel sum)"=sgl 10.0 ("Divider"), "error in (no error)"=w130, "Image Src"=w127) -> ("error out"=w140:errorcluster, "Image Dst Out"=w139:T9)  [unwired: 3 in, 3 out]
            n23 = case shown="\"Range 1\", Default" w111 {
              tunnel: ["Range 1 Templates - LEFT" "Range 0 Templates" "Range 2 Templates" "Range 3 Templates"] -> w172
              tunnel: [w538 w546 w558 w565] -> w170
              tunnel: [sgl 2.0 sgl 0.0 sgl 5.0 sgl 5.0] -> w169
              tunnel: [1 1 3 3] -> w168
              tunnel: [w535 w550 w554 w563] -> w113
              tunnel: "Correlation Score Threhsold" -> [w535 _ w554 w563]
              tunnel: "Correlation Score Threhsold (Range 0)" -> [_ w550 _ _]
              tunnel: [w533 w544 w552 w561] -> w108
              tunnel: [w532 w542 w551 w560] -> w107
              frame "Range 1", Default {
                w540 = FALSE
                w539 = TRUE
                n24 = Unbundle By Name("Range 1 Default\nSetting Values") -> ("Max Scale Diff\nfrom Main"=w533:dbl, "Beacon Cushion (px)"=w532:dbl)
                n25 = Build Array(w539, w539, w540, w540, w540) -> (w538:bool[])
              }
              frame "Range 0" {
                (unwired) TRUE
                w547 = FALSE
                n26 = Unbundle By Name("Range 0 Default\nSetting Values") -> ("Max Scale Diff\nfrom Main"=w544:dbl, "Beacon Cushion (px)"=w542:dbl)
                n27 = Build Array(w547, w547, w547, w547, w547) -> (w546:bool[])
              }
              frame "Range 2" {
                (unwired) FALSE
                w559 = TRUE
                n28 = Unbundle By Name("Range 2 Default\nSetting Values") -> ("Max Scale Diff\nfrom Main"=w552:dbl, "Beacon Cushion (px)"=w551:dbl)
                n29 = Build Array(w559, w559, w559, w559, w559) -> (w558:bool[])
              }
              frame "Range 3" {
                (unwired) FALSE
                w566 = TRUE
                n30 = Unbundle By Name("Range 3 Default\nSetting Values") -> ("Max Scale Diff\nfrom Main"=w561:dbl, "Beacon Cushion (px)"=w560:dbl)
                n31 = Build Array(w566, w566, w566, w566, w566) -> (w565:bool[])
              }
            }
            n32 = Unbundle(w172) -> ("Sub - 2 File Path"=w124:path, "Sub Beacon Template File Path - ARRAY"=w171:path[])
            n33 = call "pattern_match_subvi.vi"("Match Image In"=w139, "Settings"=w123, "Template Image In"=w122, "select (false=mod))"="select (true= use advanced features\nfase= dont use)", "ROI Descriptor"=w125, "error in (no error)"=w140, "Path In"=w124) -> ("Refnum out"=w119:T9, "Number of Matches"=w120:i32, "Matches"=w121:T13[], "error out"=w118:errorcluster)  [unwired: 5 in]
            n34 = Equal?(x=w120, y=1) -> (x = y?=w177:bool)
            n35 = Array To Cluster(array=w121) -> (cluster=w176:T14)
            n36 = Unbundle By Name(w176) -> ("Matches[0].Correlation Score"=w175:sgl)
            "Current Correlation Score" <- w175
            n37 = Greater?(x=w175, y=w113) -> (0:w174:bool)
            n38 = And(x=w177, y=w174) -> (x .and. y?=w173:bool)
            n39 = case shown="True" w173 {
              tunnel: w119 -> [w645 w673]
              tunnel: w169 -> [_ w675]
              tunnel: w170 -> [_ w674]
              tunnel: w118 -> [_ w672]
              tunnel: w123 -> [_ w671]
              tunnel: [w650 w660] -> w184
              tunnel: [w649 w670] -> w183
              tunnel: [w649 w669] -> w182
              tunnel: [w649 w659] -> w181
              tunnel: [w649 w668] -> w226
              tunnel: [w648 w657] -> w221
              tunnel: [w648 w658] -> w220
              tunnel: [w645 w667] -> w190
              tunnel: [w646 w663] -> w110
              tunnel: w176 -> [_ w666]
              tunnel: w171 -> [_ w665]
              tunnel: w111 -> [_ w664]
              tunnel: [w642 w662] -> w109
              tunnel: w108 -> [_ w656]
              tunnel: w107 -> [_ w655]
              frame False {
                w647 = 0.0
                w648 = sgl 0.0 ("Scale")
                # "Don't Move servo"
                n40 = Bundle(w647, w647) -> (w646:cluster{dbl, dbl})  [unwired: 1 in]
                n41 = Bundle(159.0, 119.0) -> (w642:cluster{dbl, dbl})  [unwired: 1 in]
                n42 = Initialize Array(FALSE, 5 ("dimension size")) -> (w650:bool[])
                n43 = Initialize Array(0.0, 5 ("dimension size")) -> (w649:dbl[])
              }
              frame True {
                n44 = Unbundle By Name(w666) -> ("Matches[0].Position"=w663:cluster{"x":sgl, "y":sgl}, "Matches[0].Bounding Box"=w676:cluster{"x":sgl, "y":sgl}[], "Matches[0].Scale"=w657:sgl, "Matches[0].Score"=w658:sgl)
                n45 = case shown="\"Range 1\", Default" w664 {
                  tunnel: w676 -> [w720 _]
                  tunnel: w675 -> [w716 _]
                  tunnel: w674 -> [w704 _]
                  tunnel: w673 -> [w702 w775]
                  tunnel: w672 -> [w701 _]
                  tunnel: w671 -> [w700 _]
                  tunnel: [w698 w784] -> w661
                  tunnel: [w697 w778] -> w670
                  tunnel: [w696 w779] -> w669
                  tunnel: [w695 w780] -> w659
                  tunnel: [w694 w781] -> w668
                  tunnel: w657 -> [w693 _]
                  tunnel: [w692 w775] -> w667
                  tunnel: w665 -> [w691 _]
                  tunnel: w657 -> [_ w776]
                  tunnel: [w690 w772] -> w662
                  tunnel: w663 -> [w690 _]
                  tunnel: w655 -> [w689 _]
                  frame "Range 1", Default {
                    # "Build ROI for Individual Beacons Based on Main Bounding Box"
                    # "Starting X Lower Bound"
                    # "Beacons to Search For"
                    # "Length of\nIndividual Beacon ROI"
                    # "Length of Bounding Box"
                    # "Draw Bounding Box on Display Image"
                    n46 = Array To Cluster(array=w720) -> (cluster=w721:T15)
                    n47 = Unbundle By Name(w721) -> ("Bounding Box[0].x"=w714:sgl, "Bounding Box[0].y"=w711:sgl, "Bounding Box[2].x"=w717:sgl, "Bounding Box[2].y"=w710:sgl)
                    n48 = Bundle("x"=w714, "y"=w711, "x"=w717, "y"=w710) -> (w719:cluster{"x":sgl, "y":sgl, "x":sgl, "y":sgl})  [unwired: 1 in]
                    n49 = call "IMAQ Overlay Rectangle"("Rectangle"=w719, "Image"=w702) -> ("Image Out"=w699:T9)  [unwired: 8 in, 1 out]
                    n50 = Subtract(x=w717, y=w714) -> (x-y=w718:sgl)
                    n51 = Divide(x=w718, y=w716) -> (x/y=w715:sgl)
                    n52 = Multiply(x=w689, y=w693) -> (x*y=w712:dbl)
                    n53 = Divide(x=w712, y=sgl 100.0) -> (x/y=w707:dbl)
                    n54 = Subtract(x=w711, y=w707) -> (x-y=w709:dbl)
                    n55 = Add(x=w710, y=w707) -> (x+y=w708:dbl)
                    n56 = for {
                      N: 5 -> [_]
                      tunnel: w704 -> [w767] mode=indexing
                      shift-right: [w761] -> _
                      shift-left: w714 -> [w766]
                      tunnel: w715 -> [w765]
                      tunnel: w709 -> [w758]
                      tunnel: w708 -> [w757]
                      tunnel: [w764] -> w703 mode=indexing
                      tunnel: w707 -> [w759]
                      # "Divide Bounding Box"
                      # "Upper Bound of Current is\nLower Bound for Next"
                      n57 = case shown="True" w767 {
                        tunnel: w766 -> [w768 w769]
                        tunnel: w765 -> [_ w771]
                        tunnel: [w768 w770] -> w761
                        tunnel: [w768 w769] -> w763
                        frame False {
                          # "Don't Care"
                        }
                        frame True {
                          # "X Lower Bound"
                          n58 = Add(x=w769, y=w771) -> (x+y=w770:sgl)
                        }
                      }
                      n59 = Subtract(x=w763, y=w759) -> (x-y=w762:dbl)
                      n60 = Add(x=w761, y=w759) -> (x+y=w760:dbl)
                      n61 = call "Bound_RO_R_R0I.vi"("Bottom Right - Y"=w757, "Right - X"=w760, "Top Left - Y"=w758, "Top  Left - x"=w762) -> ("ROI Descriptor"=w764:T12)  [unwired: 7 in]
                    }
                    n62 = for {
                      N: 5 -> [_]
                      tunnel: w702 -> [w734]
                      tunnel: w701 -> [w733]
                      tunnel: w703 -> [w726] mode=indexing
                      tunnel: w691 -> [w732] mode=indexing
                      tunnel: [w731] -> w697 mode=indexing
                      tunnel: [w730] -> w696 mode=indexing
                      tunnel: [w729] -> w698 mode=indexing
                      tunnel: w704 -> [w728] mode=indexing
                      tunnel: w700 -> [w727]
                      shift-right: [w724] -> w692
                      shift-left: w699 -> [w725]
                      tunnel: [w723] -> w695 mode=indexing
                      tunnel: [w722] -> w694 mode=indexing
                      n63 = case shown="True" w728 {
                        tunnel: w734 -> [_ w749]
                        tunnel: w733 -> [_ w748]
                        tunnel: w726 -> [_ w747]
                        tunnel: w732 -> [_ w746]
                        tunnel: [w735 w742] -> w731
                        tunnel: [w735 w741] -> w730
                        tunnel: [FALSE w740] -> w729
                        tunnel: w727 -> [_ w739]
                        tunnel: [w735 w738] -> w723
                        tunnel: [w735 w737] -> w722
                        frame False {
                          w735 = sgl 0.0 ("x")
                        }
                        frame True {
                          n64 = call "Sub Beacon Pattern Match"("Image In"=w749, "ROI Descriptor (Geometric Matching 1)"=w747, "Settings (Geometric Matching 1)"=w739, "Template File Path (Geometric Matching 1)"=w746, "error in"=w748) -> ("Matches (Geometric Matching 1)"=w743:T13[], "Number of Matches (Geometric Matching 1)"=w744:i32)  [unwired: 19 in, 2 out]
                          n65 = Equal?(x=w744, y=1) -> (x = y?=w740:bool)
                          n66 = case shown="True" w740 {
                            tunnel: w743 -> [_ w755]
                            tunnel: [w750 w754] -> w742
                            tunnel: [w750 w753] -> w741
                            tunnel: [w750 w752] -> w738
                            tunnel: [w750 w751] -> w737
                            frame False {
                              w750 = sgl 0.0 ("x")
                            }
                            frame True {
                              n67 = Array To Cluster(array=w755) -> (cluster=w756:T16)
                              n68 = Unbundle By Name(w756) -> ("Matches (Geometric Matching 1)[0].Position.x"=w754:sgl, "Matches (Geometric Matching 1)[0].Position.y"=w753:sgl, "Matches (Geometric Matching 1)[0].Scale"=w752:sgl, "Matches (Geometric Matching 1)[0].Score"=w751:sgl)
                            }
                          }
                        }
                      }
                      n69 = call "IMAQ Overlay ROI"("ROI Descriptor"=w726, "Image"=w725) -> ("Image Out"=w724:T9)  [unwired: 8 in, 1 out]
                    }
                    "Horiztonall Beacon \nCushion (pixels)" <- w689
                  }
                  frame "Range 0" {
                    w777 = sgl 0.0
                    w783 = FALSE
                    # "Don't Move servo"
                    # "Insert Current Scale into index 0"
                    n70 = Bundle(159.0, 119.0) -> (w772:cluster{dbl, dbl})  [unwired: 1 in]
                    n71 = Build Array(TRUE, w783, w783, w783, w783) -> (w784:bool[])
                    n72 = Build Array(w776, w777, w777, w777, w777) -> (w780:sgl[])
                    n73 = Build Array(w777, w777, w777, w777, w777) -> (w779:sgl[])
                    n74 = Build Array(w777, w777, w777, w777, w777) -> (w781:sgl[])
                    n75 = Build Array(w777, w777, w777, w777, w777) -> (w778:sgl[])
                  }
                }
                n76 = for {
                  tunnel: w657 -> [w681]
                  tunnel: w661 -> [w680] mode=indexing
                  tunnel: [w679] -> w660 mode=indexing
                  tunnel: w659 -> [w678] mode=indexing
                  tunnel: w656 -> [w677]
                  # "Check if Scale is within threshold of main,\ndsicard if not"
                  n77 = case shown="True" w680 {
                    selector: w680 -> [w682 _]
                    tunnel: w678 -> [_ w688]
                    tunnel: w681 -> [_ w687]
                    tunnel: [w682 w684] -> w679
                    tunnel: w677 -> [_ w683]
                    frame False {
                    }
                    frame True {
                      n78 = Subtract(x=w688, y=w687) -> (x-y=w686:sgl)
                      n79 = Absolute Value(x=w686) -> (abs(x)=w685:sgl)
                      n80 = Less?(x=w685, y=w683) -> (x < y?=w684:bool)
                    }
                  }
                }
              }
            }
            "Beacons Found" <- w184
            "X Coordinates" <- w183
            "Y Coordinates" <- w182
            "Beacon - Scales" <- w181
            "beacon - Scores" <- w226
            "Current  Scale" <- w221
            "Current  Score" <- w220
            n81 = shared-variable "RT myRIO Target - Overlord\\Localization_Variables_r0.lvlib\\LEFT_BEACON_BOOL_array"(w184) -> ()  [unwired: 1 in, 1 out]
            n82 = shared-variable "RT myRIO Target - Overlord\\Localization_Variables_r0.lvlib\\LEFT_BEACON_X_array"(w183) -> ()  [unwired: 1 in, 1 out]
            n83 = shared-variable "RT myRIO Target - Overlord\\Localization_Variables_r0.lvlib\\LEFT_BEACON_Y_array"(w182) -> ()  [unwired: 1 in, 1 out]
            n84 = shared-variable "RT myRIO Target - Overlord\\Localization_Variables_r0.lvlib\\LEFT_BEACON_Scales"(w181) -> ()  [unwired: 1 in, 1 out]
            n85 = Boolean To (0,1)(Boolean=w184) -> (0, 1=w228:i16[])
            n86 = Add Array Elements(numeric array=w228) -> (sum=w227:i16)
            n87 = Greater Or Equal?(x=w227, y=w168) -> (x >= y?=w159:bool)
            "Current Valid?" <- w159
            n88 = local read "History Size"() -> (w212:i32)
            n89 = Decrement(x=w212) -> (x-1=w225:i32)
            n90 = for {
              N: w212 -> [_]
              shift-right: [w620] -> w179
              shift-left: w224 -> [w608]
              tunnel: w225 -> [w616]
              shift-right: [w613] -> w147
              shift-left: w223 -> [w615]
              shift-right: [w612] -> w178
              shift-left: w222 -> [w614]
              tunnel: w221 -> [w611]
              tunnel: w220 -> [w610]
              tunnel: w159 -> [w609]
              i -> [w619]
              # "Reverse Index"
              n91 = Subtract(x=w616, y=w619) -> (x-y=w617:i32)
              n92 = Equal To 0?(x=w617) -> (x = 0?=w618:bool)
              n93 = case shown="True" w618 {
                tunnel: w617 -> [w621 w640]
                tunnel: w608 -> [w631 w633]
                tunnel: [w629 w632] -> w620
                tunnel: w609 -> [_ w641]
                tunnel: w615 -> [w626 w639]
                tunnel: w614 -> [w625 w638]
                tunnel: [w624 w636] -> w613
                tunnel: [w623 w637] -> w612
                tunnel: w611 -> [_ w635]
                tunnel: w610 -> [_ w634]
                frame False {
                  # "Shift Old"
                  n94 = Decrement(x=w621) -> (x-1=w622:i32)
                  n95 = Index Array(array=w631, index=w622) -> (element=w630:bool)
                  n96 = Index Array(array=w626, index=w622) -> (element=w628:dbl)
                  n97 = Index Array(array=w625, index=w622) -> (element=w627:dbl)
                  n98 = Replace Array Subset(array=w631, new element=w630, index=w621) -> (w629:bool[])
                  n99 = Replace Array Subset(array=w626, new element=w628, index=w621) -> (w624:dbl[])
                  n100 = Replace Array Subset(array=w625, new element=w627, index=w621) -> (w623:dbl[])
                }
                frame True {
                  # "Score"
                  # "Scale"
                  # "Valid"
                  # "insert New"
                  n101 = Replace Array Subset(array=w639, new element=w635, index=w640) -> (w636:dbl[])
                  n102 = Replace Array Subset(array=w638, new element=w634, index=w640) -> (w637:dbl[])
                  n103 = Replace Array Subset(array=w633, new element=w641, index=w640) -> (w632:bool[])
                }
              }
            }
            n104 = Boolean To (0,1)(Boolean=w179) -> (0, 1=w218:i16[])
            n105 = Add Array Elements(numeric array=w218) -> (sum=w217:i16)
            n106 = Greater Or Equal?(x=w217, y="Valid Treshold\nfor Lock") -> (x >= y?=w145:bool)
            "Lock Status" <- w145
            n107 = shared-variable "RT myRIO Target - Overlord\\Localization_Variables_r0.lvlib\\Image Lock - L"(w145) -> ()  [unwired: 1 in, 1 out]
            n108 = Initialize Array(u8 0, "Max Window\n for Avg") -> (w215:u8[])
            n109 = while {
              shift-right: [w591] -> w211
              shift-left: w215 -> [w593]
              tunnel: w179 -> [w599] mode=indexing
              shift-right: [w597] -> w208
              shift-left: u8 0 -> [w600]
              tunnel: w212 -> [w598]
              tunnel: "Max Window\n for Avg" -> [w590]
              i -> [w592]
              stop <- w594 stop-if-true
              # "Grab Last 'X' Valid Indexes"
              n110 = case shown="True" w599 {
                tunnel: w600 -> [w602 w604]
                tunnel: [w602 w607] -> w597
                tunnel: w593 -> [w601 w606]
                tunnel: w592 -> [_ w605]
                tunnel: [w601 w603] -> w591
                frame False {
                }
                frame True {
                  # "Update Index\nto use"
                  # "Increment\nValid Count"
                  n111 = Replace Array Subset(array=w606, new element=w605, index=w604) -> (w603:u8[])
                  n112 = Increment(x=w604) -> (x+1=w607:u8)
                }
              }
              n113 = Greater?(x=w592, y=w598) -> (0:w595:bool)
              n114 = Greater Or Equal?(x=w597, y=w590) -> (x >= y?=w596:bool)
              n115 = Or(x=w596, y=w595) -> (x .or. y?=w594:bool)
            }
            n116 = Greater Or Equal?(x=w208, y=u8 2) -> (x >= y?=w209:bool)
            n117 = case shown="True" w209 {
              tunnel: w208 -> [_ w574]
              tunnel: w211 -> [_ w580]
              tunnel: w147 -> [_ w579]
              tunnel: w178 -> [_ w578]
              tunnel: ["Avg Scale - Last" w572] -> w167
              tunnel: ["Avg Score - Last" w571] -> w166
              frame False {
              }
              frame True {
                w577 = 0.0
                n118 = for {
                  N: w574 -> [_]
                  tunnel: w580 -> [w587] mode=indexing
                  tunnel: w579 -> [w589]
                  tunnel: w578 -> [w588]
                  shift-right: [w585] -> w576
                  shift-left: w577 -> [w583]
                  shift-right: [w586] -> w575
                  shift-left: w577 -> [w582]
                  # "Fetch Last Valid Values"
                  n119 = Index Array(array=w589, index=w587) -> (element=w584:dbl)
                  n120 = Index Array(array=w588, index=w587) -> (element=w581:dbl)
                  n121 = Add(x=w584, y=w583) -> (x+y=w585:dbl)
                  n122 = Add(x=w581, y=w582) -> (x+y=w586:dbl)
                }
                n123 = To Double Precision Float(number=w574) -> (double precision float=w573:dbl)
                n124 = Divide(x=w576, y=w573) -> (x/y=w572:dbl)
                n125 = Divide(x=w575, y=w573) -> (x/y=w571:dbl)
                n126 = local write "Avg Scale - Last"(w572) -> ()
                n127 = local write "Avg Score - Last"(w571) -> ()
              }
            }
            "Avg Score" <- w166
            "Avg Scale" <- w167
            n128 = And(x=w145, y=w144) -> (x .and. y?=w146:bool)
            n129 = case shown="False" w146 {
              selector: w146 -> [_ w232]
              tunnel: [w230 w231] -> w143
              tunnel: w144 -> [w230 _]
              frame False {
              }
              frame True {
                # "Pull Down Start Up \nFlag"
                n130 = Not(x=w232) -> (.not. x?=w231:bool)
              }
            }
            n131 = Unbundle By Name(w123) -> ("Minimum Match Score"=w164:sgl, "Range Settings"=w195:T7[], "Curve Parameters"=w161:T6)
            n132 = Index Array(array=w195, index=u32 1) -> (element=w196:T7)
            n133 = Unbundle(w196) -> ("Min"=w163:dbl, "Max"=w162:dbl)  [unwired: 1 out]
            n134 = case shown="False" w143 {
              tunnel: w145 -> [w255 _]
              tunnel: w111 -> [w254 w531]
              tunnel: w167 -> [w253 _]
              tunnel: [w237 w531] -> w149
              tunnel: w167 -> [w252 _]
              tunnel: w166 -> [w251 _]
              tunnel: "Score\nCushion" -> [w250 _]
              tunnel: w164 -> [w249 w528]
              tunnel: w163 -> [w248 w527]
              tunnel: w162 -> [w247 w526]
              tunnel: w110 -> [w246 _]
              tunnel: w125 -> [w245 w530]
              tunnel: w161 -> [w244 _]
              tunnel: w161 -> [w243 w529]
              tunnel: [w242 w528] -> w153
              tunnel: [w241 w527] -> w151
              tunnel: [w240 w526] -> w152
              tunnel: [w239 w530] -> w150
              tunnel: [w238 w529] -> w158
              tunnel: [w236 FALSE] -> w160
              tunnel: w159 -> [w235 _]
              tunnel: w147 -> [w234 w524]
              tunnel: [w233 w524] -> w148
              frame False {
                # "Current Template"
                # "Image Lock?"
                n135 = case shown="True" w255 {
                  tunnel: w254 -> [w281 w323]
                  tunnel: [w281 w286] -> w237
                  tunnel: w253 -> [_ w324]
                  tunnel: w252 -> [_ w322]
                  tunnel: w251 -> [_ w320]
                  tunnel: w250 -> [_ w319]
                  tunnel: w249 -> [_ w318]
                  tunnel: w248 -> [_ w317]
                  tunnel: w247 -> [_ w316]
                  tunnel: w246 -> [_ w315]
                  tunnel: w245 -> [_ w314]
                  tunnel: w244 -> [_ w311]
                  tunnel: w243 -> [w259 w296]
                  tunnel: [w258 w291] -> w238
                  tunnel: [w270 w290] -> w239
                  tunnel: [w279 w289] -> w242
                  tunnel: [w278 w288] -> w241
                  tunnel: [w277 w287] -> w240
                  tunnel: [FALSE w285] -> w236
                  tunnel: w235 -> [_ w284]
                  tunnel: w234 -> [w256 w283]
                  tunnel: [w256 w282] -> w233
                  frame False {
                    # "Initial ROI Descriptor"
                    # "Check Other Camera?"
                    n136 = Unbundle By Name("No Lock Default\nSetting Values") -> ("Min Score"=w279:dbl, "Min Scale"=w278:dbl, "Max Scale"=w277:dbl, "Curve Parameters"=w260:T17)
                    n137 = Bundle(0, 0, 640, 480, 0) -> (w276:cluster{i32, i32, i32, i32, i32})  [unwired: 1 in]
                    n138 = call "IMAQ Convert Rectangle to ROI"("Rectangle"=w276) -> ("ROI Descriptor"=w270:T12)  [unwired: 8 in, 1 out]
                    n139 = Unbundle By Name(w260) -> ("Min Length"=w264:i32, "Row Search Step"=w265:i32, "Col Search Step"=w266:i32)
                    n140 = Unbundle(w259) -> ("Extraction Mode"=w261:u32, "Edge Threshold"=w262:i32, "Edge Filter Size"=w263:u32, "Max Endpoint Gap"=w267:i32, "Closed"=w268:bool, "Subpixel"=w269:bool)  [unwired: 3 out]
                    n141 = Bundle("Extraction Mode"=w261, "Edge Threshold"=w262, "Edge Filter Size"=w263, "Min Length"=w264, "Row Search Step"=w265, "Col Search Step"=w266, "Max Endpoint Gap"=w267, "Closed"=w268, "Subpixel"=w269) -> (w258:T18)  [unwired: 1 in]
                  }
                  frame True {
                    # "Update Search Settings"
                    # "Next State"
                    # "Changing Templates?"
                    # "Update Template"
                    n142 = case shown="\"Range 1\", Default" w323 {
                      selector: w323 -> [w456 w487 w505 w520]
                      tunnel: w324 -> [w457 w489 w506 w521]
                      tunnel: [w458 w488 w504 w519] -> w286
                      tunnel: [w472 w478 w498 w513] -> w321
                      tunnel: [w471 w477 w497 w512] -> w313
                      tunnel: [w470 w476 w496 w511] -> w312
                      tunnel: [w469 w479 w502 w517] -> w307
                      tunnel: [w468 w481 w499 w514] -> w299
                      tunnel: [w467 w482 w500 w515] -> w298
                      tunnel: [w466 w485 w501 w516] -> w297
                      frame "Range 1", Default {
                        # "Next Template"
                        # "Next Template"
                        n143 = local read "Range 1 Default\nSetting Values"() -> (w473:T1)
                        n144 = Unbundle By Name(w473) -> ("Lower Transition Scale"=w454:sgl, "Upper Transition Scale"=w455:sgl, "ROI Vertical"=w470:dbl, "ROI Horizontal"=w471:dbl, "Scale Cushion"=w472:dbl, "Curve Parameters"=w469:T17, "Min Score"=w468:dbl, "Min Scale"=w467:dbl, "Max Scale"=w466:dbl)
                        n145 = Less?(x=w457, y=w454) -> (x < y?=w465:bool)
                        n146 = Not(x=w465) -> (.not. x?=w464:bool)
                        n147 = Select(t=w456, s=w464, f=T4."Range 2" ("Initial Template 2")) -> (s? t:f=w461:T4)
                        n148 = Greater?(x=w457, y=w455) -> (0:w463:bool)
                        n149 = Not(x=w463) -> (.not. x?=w462:bool)
                        n150 = Select(t=w461, s=w462, f=T4."Range 0" ("Initial Template 2")) -> (s? t:f=w458:T4)
                      }
                      frame "Range 2" {
                        # "Next Template"
                        # "Next Template"
                        n151 = local read "Range 2 Default\nSetting Values"() -> (w486:T1)
                        n152 = Unbundle By Name(w486) -> ("Lower Transition Scale"=w484:sgl, "Upper Transition Scale"=w483:sgl, "ROI Vertical"=w476:dbl, "ROI Horizontal"=w477:dbl, "Scale Cushion"=w478:dbl, "Curve Parameters"=w479:T17, "Min Score"=w481:dbl, "Min Scale"=w482:dbl, "Max Scale"=w485:dbl)
                        n153 = Less?(x=w489, y=w484) -> (x < y?=w493:bool)
                        n154 = Not(x=w493) -> (.not. x?=w492:bool)
                        n155 = Select(t=w487, s=w492, f=T4."Range 3" ("Initial Template 2")) -> (s? t:f=w480:T4)
                        n156 = Greater?(x=w489, y=w483) -> (0:w491:bool)
                        n157 = Not(x=w491) -> (.not. x?=w490:bool)
                        n158 = Select(t=w480, s=w490, f=T4."Range 1" ("Initial Template 2")) -> (s? t:f=w488:T4)
                      }
                      frame "Range 3" {
                        # "Next Template"
                        n159 = local read "Range 3 Default\nSetting Values"() -> (w503:T1)
                        n160 = Unbundle By Name(w503) -> ("Upper Transition Scale"=w495:sgl, "ROI Vertical"=w496:dbl, "ROI Horizontal"=w497:dbl, "Scale Cushion"=w498:dbl, "Curve Parameters"=w502:T17, "Min Score"=w499:dbl, "Min Scale"=w500:dbl, "Max Scale"=w501:dbl)  [unwired: 1 out]
                        n161 = Greater?(x=w506, y=w495) -> (0:w508:bool)
                        n162 = Not(x=w508) -> (.not. x?=w507:bool)
                        n163 = Select(t=w505, s=w507, f=T4."Range 2" ("Initial Template 2")) -> (s? t:f=w504:T4)
                      }
                      frame "Range 0" {
                        # "Next Template"
                        n164 = local read "Range 0 Default\nSetting Values"() -> (w518:T1)
                        n165 = Unbundle By Name(w518) -> ("Lower Transition Scale"=w509:sgl, "ROI Vertical"=w511:dbl, "ROI Horizontal"=w512:dbl, "Scale Cushion"=w513:dbl, "Curve Parameters"=w517:T17, "Min Score"=w514:dbl, "Min Scale"=w515:dbl, "Max Scale"=w516:dbl)  [unwired: 1 out]
                        n166 = Less?(x=w521, y=w509) -> (x < y?=w523:bool)
                        n167 = Not(x=w523) -> (.not. x?=w522:bool)
                        n168 = Select(t=w520, s=w522, f=T4."Range 1" ("Initial Template 2")) -> (s? t:f=w519:T4)
                      }
                    }
                    n169 = Unbundle By Name(w307) -> ("Min Length"=w306:i32, "Row Search Step"=w305:i32, "Col Search Step"=w304:i32)
                    n170 = Unbundle(w311) -> ("Extraction Mode"=w310:u32, "Edge Threshold"=w309:i32, "Edge Filter Size"=w308:u32, "Max Endpoint Gap"=w303:i32, "Closed"=w302:bool, "Subpixel"=w301:bool)  [unwired: 3 out]
                    n171 = Bundle("Extraction Mode"=w310, "Edge Threshold"=w309, "Edge Filter Size"=w308, "Min Length"=w306, "Row Search Step"=w305, "Col Search Step"=w304, "Max Endpoint Gap"=w303, "Closed"=w302, "Subpixel"=w301) -> (w300:T18)  [unwired: 1 in]
                    n172 = Not Equal?(x=w286, y=w323) -> (x != y?=w285:bool)
                    n173 = case shown="True" w285 {
                      tunnel: w284 -> [w347 _]
                      tunnel: w322 -> [w346 _]
                      tunnel: w321 -> [w345 _]
                      tunnel: w320 -> [w344 _]
                      tunnel: w319 -> [w343 _]
                      tunnel: w318 -> [w342 _]
                      tunnel: w317 -> [w341 _]
                      tunnel: w316 -> [w340 _]
                      tunnel: w315 -> [w339 _]
                      tunnel: w314 -> [w338 _]
                      tunnel: w313 -> [w337 _]
                      tunnel: w312 -> [w336 _]
                      tunnel: [w334 w421] -> w289
                      tunnel: w300 -> [w325 _]
                      tunnel: [w333 w420] -> w288
                      tunnel: [w332 w419] -> w287
                      tunnel: w299 -> [_ _]
                      tunnel: w298 -> [_ _]
                      tunnel: w297 -> [_ _]
                      tunnel: w286 -> [_ w423]
                      tunnel: w296 -> [_ w436]
                      tunnel: [w326 w435] -> w291
                      tunnel: [w331 w430] -> w295
                      tunnel: [w330 w429] -> w294
                      tunnel: [w329 w412] -> w293
                      tunnel: [w328 w413] -> w292
                      tunnel: w283 -> [w327 w415]
                      tunnel: [w327 w414] -> w282
                      frame False {
                        w335 = 500.0 ("y")
                        # "Current Valid?"
                        # "********"
                        # "Apply Limit to Score"
                        # "Score out"
                        # "Apply Limits to ROI"
                        n174 = case shown="False" w347 {
                          tunnel: w344 -> [_ w396]
                          tunnel: w343 -> [_ w395]
                          tunnel: w346 -> [_ w386]
                          tunnel: w345 -> [w375 w394]
                          tunnel: [w358 w389] -> w331
                          tunnel: [w357 w385] -> w330
                          tunnel: [w356 w388] -> w329
                          tunnel: [w355 w387] -> w328
                          tunnel: [w371 w384] -> w348
                          tunnel: [w370 w383] -> w333
                          tunnel: [w369 w382] -> w332
                          tunnel: w338 -> [w367 _]
                          tunnel: w342 -> [w354 _]
                          tunnel: w341 -> [w353 _]
                          tunnel: w340 -> [w352 _]
                          tunnel: w339 -> [_ w381]
                          tunnel: w337 -> [_ w377]
                          tunnel: w336 -> [_ w378]
                          tunnel: [w350 w376] -> w326
                          tunnel: w325 -> [w350 w376]
                          frame False {
                            # "Current Match was Invalid"
                            n175 = Divide(x=w375, y=sgl 3.0) -> (x/y=w373:dbl)
                            n176 = Subtract(x=w353, y=w373) -> (x-y=w370:dbl)
                            n177 = Add(x=w352, y=w373) -> (x+y=w369:dbl)
                            n178 = Subtract(x=w354, y="Score Decay \nFactor 2") -> (x-y=w371:dbl)
                            n179 = call "IMAQ Convert ROI to Rectangle"("ROI Descriptor"=w367) -> ("Rectangle"=w368:T19)  [unwired: 8 in, 1 out]
                            n180 = Unbundle By Name(w368) -> ("Left"=w362:i32, "Top"=w361:i32, "Right"=w360:i32, "Bottom"=w359:i32)
                            n181 = To Long Integer(number="ROI Decay Factor (px)") -> (32bit integer=w364:i32)
                            n182 = Divide(x="ROI Decay Factor (px)", y=sgl 10.0) -> (x/y=w366:dbl)
                            n183 = Subtract(x=w362, y=w364) -> (x-y=w358:i32)
                            n184 = Add(x=w360, y=w364) -> (x+y=w356:i32)
                            n185 = To Long Integer(number=w366) -> (32bit integer=w363:i32)
                            n186 = Subtract(x=w361, y=w363) -> (x-y=w357:i32)
                            n187 = Add(x=w359, y=w363) -> (x+y=w355:i32)
                          }
                          frame True {
                            (unwired) sgl 109.0 ("x")
                            (unwired) sgl 159.0 ("x")
                            # "Current Match was Valid"
                            # "Center of Image"
                            # "Main ROI"
                            # "Horizontal Scale \n(smaller number = smaller ROI)"
                            n188 = Subtract(x=w396, y=w395) -> (x-y=w384:dbl)
                            n189 = case shown="0, Default" "ROBOT STATE\n(fwd, bwd, neither) 2" {
                              tunnel: w386 -> [w401 w406 w411]
                              tunnel: [w400 w402 w407] -> w382
                              tunnel: w394 -> [w398 w405 w410]
                              tunnel: [w399 w403 w408] -> w383
                              frame 0, Default {
                                n190 = Subtract(x=w401, y=w398) -> (x-y=w399:dbl)
                                n191 = Add(x=w398, y=w401) -> (x+y=w400:dbl)
                              }
                              frame 1 {
                                n192 = Subtract(x=w406, y=5.0) -> (x-y=w403:dbl)
                                n193 = Add(x=w405, y=w406) -> (x+y=w402:dbl)
                              }
                              frame -1 {
                                n194 = Subtract(x=w411, y=w410) -> (x-y=w408:dbl)
                                n195 = Add(x=5.0 ("y"), y=w411) -> (x+y=w407:dbl)
                              }
                            }
                            n196 = Unbundle(w381) -> ("x"=w380:dbl, "y"=w379:dbl)
                            n197 = Divide(x=w386, y=w378) -> (x/y=w392:dbl)
                            n198 = Multiply(x=w386, y=w377) -> (x*y=w390:dbl)
                            n199 = Divide(x=w390, y=sgl 2.0) -> (x/y=w393:dbl)
                            n200 = Add(x=w379, y=w392) -> (x+y=w387:dbl)
                            n201 = Subtract(x=w379, y=w392) -> (x-y=w385:dbl)
                            n202 = Subtract(x=w380, y=w393) -> (x-y=w389:dbl)
                            n203 = Add(x=w393, y=w380) -> (x+y=w388:dbl)
                          }
                        }
                        n204 = Greater?(x=w348, y=w335) -> (0:w349:bool)
                        n205 = Select(t=w348, s=w349, f=w335) -> (s? t:f=w334:dbl)
                      }
                      frame True {
                        w416 = 80.0 ("Avg Scale - Last")
                        w426 = sgl 125.0 ("x")
                        w427 = sgl 109.0 ("x")
                        w428 = sgl 159.0 ("x")
                        # "Reset Scale to 100"
                        # "\"Start Scale\""
                        # "Center of Image"
                        # "Main ROI"
                        # "Horizontal Scale \n(smaller number = smaller ROI)"
                        # "Apply New Curve Parameters"
                        # "Next State"
                        # "Changing States - Apply Initial Settings for that State"
                        n206 = local read "History Size"() -> (w417:i32)
                        n207 = case shown="\"Range 1\", Default" w423 {
                          tunnel: [w450 w451 w452 w453] -> w422
                          frame "Range 1", Default {
                            n208 = local read "Range 1 Default\nSetting Values"() -> (w450:T1)
                          }
                          frame "Range 2" {
                            n209 = local read "Range 2 Default\nSetting Values"() -> (w451:T1)
                          }
                          frame "Range 3" {
                            n210 = local read "Range 3 Default\nSetting Values"() -> (w452:T1)
                          }
                          frame "Range 0" {
                            n211 = local read "Range 0 Default\nSetting Values"() -> (w453:T1)
                          }
                        }
                        n212 = for {
                          N: w417 -> [_]
                          tunnel: w416 -> [w447]
                          shift-right: [w446] -> w414
                          shift-left: w415 -> [w449]
                          i -> [w448]
                          n213 = Replace Array Subset(array=w449, new element=w447, index=w448) -> (w446:dbl[])
                        }
                        n214 = local write "Avg Scale - Last"(w416) -> ()
                        n215 = Unbundle By Name(w422) -> ("Min Score"=w421:dbl, "Min Scale"=w420:dbl, "Max Scale"=w419:dbl, "Curve Parameters"=w418:T17, "ROI Vertical"=w425:dbl, "ROI Horizontal"=w424:dbl)
                        n216 = Unbundle By Name(w418) -> ("Min Length"=w440:i32, "Row Search Step"=w441:i32, "Col Search Step"=w442:i32)
                        n217 = Unbundle(w436) -> ("Extraction Mode"=w437:u32, "Edge Threshold"=w438:i32, "Edge Filter Size"=w439:u32, "Max Endpoint Gap"=w443:i32, "Closed"=w444:bool, "Subpixel"=w445:bool)  [unwired: 3 out]
                        n218 = Bundle("Extraction Mode"=w437, "Edge Threshold"=w438, "Edge Filter Size"=w439, "Min Length"=w440, "Row Search Step"=w441, "Col Search Step"=w442, "Max Endpoint Gap"=w443, "Closed"=w444, "Subpixel"=w445) -> (w435:T18)  [unwired: 1 in]
                        n219 = Divide(x=w426, y=w425) -> (x/y=w433:dbl)
                        n220 = Multiply(x=w426, y=w424) -> (x*y=w431:dbl)
                        n221 = Divide(x=w431, y=sgl 2.0) -> (x/y=w434:dbl)
                        n222 = Add(x=w427, y=w433) -> (x+y=w413:dbl)
                        n223 = Subtract(x=w427, y=w433) -> (x-y=w429:dbl)
                        n224 = Subtract(x=w428, y=w434) -> (x-y=w430:dbl)
                        n225 = Add(x=w434, y=w428) -> (x+y=w412:dbl)
                      }
                    }
                    n226 = call "Bound_RO_R_R0I.vi"("Bottom Right - Y"=w292, "Right - X"=w293, "Top Left - Y"=w294, "Top  Left - x"=w295) -> ("ROI Descriptor"=w290:T12)  [unwired: 7 in]
                  }
                }
              }
              frame True {
              }
            }
            "Next Template" <- w149
            n227 = Less?(x=w153, y="Absolute\nMinimum Score") -> (x < y?=w201:bool)
            n228 = Less?(x=w151, y="Absolute\nMinimum Scale") -> (x < y?=w204:bool)
            n229 = Greater?(x=w152, y="Absolute\nMaximum Scale") -> (0:w207:bool)
            n230 = Greater?(x=w151, y=w152) -> (0:w203:bool)
            n231 = Less?(x=w152, y=w151) -> (x < y?=w206:bool)
            n232 = Select(t="Absolute\nMinimum Score", s=w201, f=w153) -> (s? t:f=w189:dbl)
            "New Min Score" <- w189
            n233 = Or(x=w204, y=w203) -> (x .or. y?=w202:bool)
            n234 = Or(x=w207, y=w206) -> (x .or. y?=w205:bool)
            n235 = Select(t="Absolute\nMinimum Scale", s=w202, f=w151) -> (s? t:f=w188:dbl)
            "New Low Scale" <- w188
            n236 = Select(t="Absolute\nMaximum Scale", s=w205, f=w152) -> (s? t:f=w187:dbl)
            "New high Scale" <- w187
            n237 = Bundle("index"=w194, "Min"=w188, "Max"=w187) -> (w193:cluster{"index":u32, "Min":dbl, "Max":dbl})  [unwired: 1 in]
            n238 = Replace Array Subset(array=w195, new element=w193, index=w194) -> (w192:T7[])
            n239 = Bundle By Name(cluster=w123, "Minimum Match Score"=w189, "Range Settings"=w192, "Curve Parameters"=w158) -> (w191:T8)
            n240 = call "IMAQ Overlay ROI"("ROI Descriptor"=w150, "Image"=w190) -> ("Image Out"=→"Right Image out":T9)  [unwired: 8 in, 1 out]
            n241 = Unbundle By Name(w158) -> ("Min Length"=w157:i32, "Row Search Step Size"=w156:i32, "Col Search Step Size"=w155:i32)
            n242 = Bundle("Min Length"=w157, "Row Search Step Size"=w156, "Col Search Step Size"=w155) -> (w154:T20)  [unwired: 1 in]
            n243 = Bundle("Min Score"=w189, "Min"=w188, "Max"=w187, w154) -> (w186:T21)  [unwired: 1 in]
            n244 = case shown="True" w160 {
              tunnel: w109 -> [w787 w793]
              tunnel: w159 -> [w788 w799]
              tunnel: w184 -> [_ _]
              tunnel: w186 -> [w790 w797]
              tunnel: w145 -> [w789 w800]
              tunnel: w149 -> [w786 w798]
              tunnel: [w785 w796] -> w142
              frame False {
                n245 = Bundle(w789, w788, "Initial Template"=w786, "Position"=w787, w790) -> (w785:T22)  [unwired: 1 in]
              }
              frame True {
                # "Check if Tracking is Available for the Next Template State"
                n246 = local read "Current Template"() -> (w791:T4)
                n247 = Unbundle(w793) -> ("x"=w795:dbl, "y"=w794:dbl)
                n248 = case shown="\"Range 1\"" w798 {
                  tunnel: w795 -> [w805 w814 _ _]
                  tunnel: w794 -> [w801 w813 _ _]
                  tunnel: w793 -> [_ w811 w822 _]
                  tunnel: [w804 w812 w822 w825] -> w792
                  tunnel: w791 -> [w802 w810 _ _]
                  frame "Range 1" {
                    n249 = case shown="\"Range 2\"" w802 {
                      tunnel: w805 -> [w806 w809]
                      tunnel: [w806 w807] -> w803
                      frame "Range 0", Default {
                      }
                      frame "Range 2" {
                        n250 = Add(x=w809, y=-70.0) -> (x+y=w807:dbl)
                      }
                    }
                    n251 = Bundle("x"=w803, "y"=w801) -> (w804:cluster{"x":dbl, "y":dbl})  [unwired: 1 in]
                  }
                  frame "Range 2" {
                    # "Depends on Current State"
                    n252 = case shown="\"Range 3\"" w810 {
                      tunnel: w814 -> [w819 _ _]
                      tunnel: w813 -> [w816 _ _]
                      tunnel: [w815 w820 w821] -> w812
                      tunnel: w811 -> [_ w820 w821]
                      frame "Range 1" {
                        n253 = Add(x=w819, y=70.0) -> (x+y=w817:dbl)
                        n254 = Bundle(w817, "y"=w816) -> (w815:cluster{dbl, "y":dbl})  [unwired: 1 in]
                      }
                      frame "Range 2", Default {
                      }
                      frame "Range 3" {
                      }
                    }
                  }
                  frame "Range 3", Default {
                  }
                  frame "Range 0" {
                    # "Don't Move servo"
                    n255 = Bundle(159.0, 119.0) -> (w825:cluster{dbl, dbl})  [unwired: 1 in]
                  }
                }
                n256 = Bundle(w800, w799, "Initial Template"=w798, "Position"=w792, w797) -> (w796:T22)  [unwired: 1 in]
              }
            }
            "Tracking Info" <- w142
            n257 = shared-variable "RT myRIO Target - Overlord\\Localization_Variables_r0.lvlib\\Info - Left"(w142) -> ()  [unwired: 1 in, 1 out]
          }
          frame #2 {
            n258 = shared-variable "RT myRIO Target - Overlord\\Localization_Variables_r0.lvlib\\Left Servo Angle_Image"(w828) -> ()  [unwired: 1 in, 1 out]
            n259 = shared-variable "RT myRIO Target - Overlord\\Localization_Variables_r0.lvlib\\Left_Flag"(TRUE ("RIGHT_FLAG")) -> ()  [unwired: 1 in, 1 out]
          }
        }
        "Startup Flag" <- w75
        "Valid Scale History" <- w82
        "Valid Beacon History - in" <- w84
        "Valid Score History" <- w81
        "Current Search Settings" <- w92
        "Current Template" <- w79
      }
    }
    frame #2 {
      n260 = call <vilib>:"IMAQdx Close Camera.vi"("Session In"=w830) -> ()  [unwired: 10 in, 1 out]
    }
  }
